vi "MonoVu.vi"() -> ()   [LabVIEW 2025]
doc: "Sequence Program with the Message Handling Queue (MHQ) for the National High Magnetic Field Laboratory in Tallahassee, Florida. \nOnce you understand how the programs works, you should be able to modify this program easily. If you have any questions, contact Minseong Lee(ml10k@my.fsu.edu), who first made this program in June, 2015."
uses:
  <vilib>/printing/OpenHTMLReport.llb/Open HTML Report in Browser (Path).vi
  <vilib>/Utility/NIReport.llb/NI_ReportGenerationCore.lvlib
panel:
  out "Row":i32=14
  in  "reset\ncursor":bool
  in  "Tab Control":T1(tab)
  in  "Sequence":i32[](listbox)=[8]
  in  "Commands":string(tree)="Remarks"
  out "Sequence Status":string="Status window"
  in  "index":i32[](listbox)=[8] caption="Sequence"
  in  "Use absolute sequence path":bool
  in  "Sequences folder path":path=path "c:/Users/user/Desktop/Sequences"
  in  "Magnet PS":u16(ring)=3 items=["Resistive Magnet", "SCM2", "SCM1", "Generic SC power supply", "PPMS"]
  in  "platform":u16(ring) items=["Mac", "PC"]
  in  "NML Data Acquisition VI":string(combo)="NML Data Acquisition-New.vi"
  in  "wait after each line executed (ms)":u32
  in  "interval in a looped execution":u32=100
  in  "PS Control VI Name":string="PS Control.vi"
  in  "override command error":bool
  in  "horizontal lines":bool
  in  "line numbers":bool
  out "most recent error":errorcluster={"status"=TRUE, "code"=1004, "source"="Open VI Reference in Get_Vi_Data.vi->WaitForAnyVI.vi->MonoVu.vi<APPEND>\nTo load a VI into memory with the Open VI Reference function, a path must be wired for the VI Path input.\n\nVI Name: <b>BLM_ManualControl.vi</b>"}
  out "execution count":i32=1
  out "macro line":i32
  out "sequence contents":string[](array[string])=["----------    AH Bridge: Set data and Time (To remove 'RTC WAS RESET' message)  ", "Write to VISA, GPIB0::27::INSTR, STORE DATE 2020,1,27", "Write to VISA, GPIB0::27::INSTR, STORE TIME 12, 45, 27", "----------    AH Bridge: Save GPIB address   ", "Write to VISA, GPIB::27::INSTR, FILE STORE GPIB USERPON", "----------    LakeShore 340 controller: change heater power (0-5, 0: off)  ", "Write to VISA, GPIB::12::INSTR, RANGE 0", "----------    Scheduled T-control for the He3 system   ", "Wait for 12 hour", "Set Temperature LS336 ( GPIB0::12::INSTR ) 45 K at 0 K/min, Output 1", "Wait for 60 s", "Wait for Temperature Less than 1.8 K Sensor C of LS336 ( GPIB0::14::INSTR ) Timeout 30 min", "Wait for 60 min", "Set Temperature LS336 ( GPIB0::12::INSTR ) 0.1 K at 0 K/min, Output 1", "----------    Motor control (use Instrumet:Set:MotorControl command structure)  ", "Set MotorControl ( BLM ) 12345 0.2", "Wait for VI value localhost, BLM_ManualControl.vi, BLM Position, Within, 12345, 10 min", "END SEQUENCE"]
  in  "error\ncheck":bool
  in  "exec window":bool caption="command window"
  in  "loop stop":bool
  in  "error \nindicator":bool
  out "Error/\nwarning?":bool
  in  "sequence utility":bool caption="seq\n utility"
  out "macro cmd no":i32=34
  in  "track \nseq.":bool
  in  "help":bool caption="Help"
  out "Buffer Edit":string[](array[string])=["----------    AH Bridge: Save GPIB address   "]
  out "Path":path=path "/Users/Shared/NML Data Acquisition/monovu/sequence templates/system typical 2.txt"
  out "Buffer History":string[](array[string])
  in  "Skip Button":bool caption="Skip"
  in  "error in (no error)":errorcluster
  in  "New Button":bool caption="New"
  in  "Program Stop":bool=TRUE caption="Program \nStop"
  in  "Save Button":bool caption="Save"
  in  "Sequence_Stop":bool caption="Stop"
  in  "Pause Button":bool caption="Pause"
  in  "Run Sequence":bool caption="Run"
  in  "Save As Button":bool caption="Save As"
  out "Cursor Position":i32=8
  out "Current Line":i32
  in  "Open Button":bool caption="Open"
  # "Timing parameters"
  # "User interface settings"
  # "Sequence Window"
  # "*"
  # "(when abs. path not used)"
  # "(bypass command syntax error)"
  # "*"
  # ": Needs to restart this VI to make the change effective"
  # "(see logbook for previous errors)"
  # "Note \n(1) For commands with timed or conditioned wait, 'go to next line' command will be executed when a certain condition is met.\n(2) For non-wait command (send command to instruments or VI without waiting response), 'go to next line' is executed automatically.\n(3) For example, 'wait for temperature command' executes repeatedly until the temperature condition is met. The visa reference will be open and closed every time it is executed.\n** Exception: 'Wait for VI value' uses a loop to use the VI reference. The loop condition has to be programmatically reset for the user intervention (skip, pause, stop) accordingly.\n\n\n\nNote for coding\n1. Each comand in the sequence line is executed repeatedly until a 'go to next line' command is executed by itself or by user interruption.\n2. 'go to next line' condition is defined in the VI of each command.\n3. Right mouse click button menu modification : Right mouse click on the sequence window -> advanced -> Run time shorcut menu -> edit"
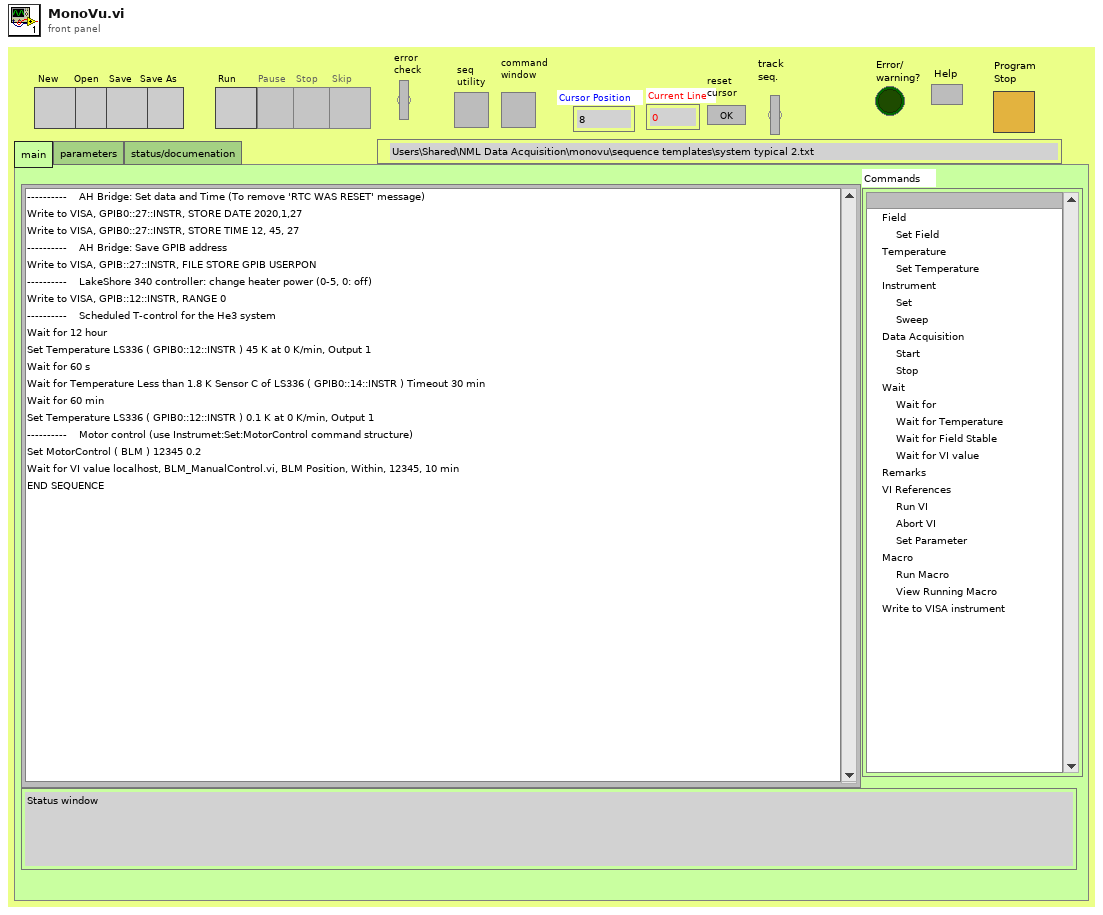
[diagram p1: front panel]
types:
  T1 = enum32{"main", "parameters", "status/documenation"}
  T2 = cluster{"Sequence_Run":refnum<vi>, "Sequence_Pause":refnum<vi>, "Sequence_Stop":refnum<vi>, "Sequence_Skip":refnum<vi>, "Program Stop":refnum<vi>, "Sequence":refnum<vi>, "NML Data Acquisition VI":refnum<vi>}
  T3 = cluster{"number of line":i32, "Signal":bool, "Command":string, "Sequence Reference":refnum<vi>, "Add or modification":bool}
  T4 = cluster{"No. of command":i32, "Parameters":string[], "Address":refnum<visa-resource-name>, "Boolean":bool, "No. of line":i32, "Initial Time":timestamp, "Current Time":timestamp, "Status":string, "Sequence Ref.":refnum<vi>, "Temp_Check":i32, "Sequence_History":string, "Subsequence":string[]}
  T5 = typedef "Command_Message.ctl" = cluster{"No. of command":i32, "Parameters":string[], "Address":refnum<visa-resource-name>, "Boolean":bool, "No. of line":i32, "Initial Time":timestamp, "Current Time":timestamp, "Status":string, "Sequence Ref.":refnum<vi>, "Temp check":i32, "Sequence_History":string, "Subsequence":string[]}
  T6 = typedef "eventsource.ctl" = u32
  T7 = typedef "Button_Reference.ctl" = cluster{"Sequence_Run":refnum<vi>, "Sequence_Pause":refnum<vi>, "Sequence_Stop":refnum<vi>, "Sequence_Skip":refnum<vi>, "Program Stop":refnum<vi>, "Sequence":refnum<vi>, "NML Data Acquisition VI":refnum<vi>}
  T8 = typedef "Command_Queue.ctl" = refnum<queue>
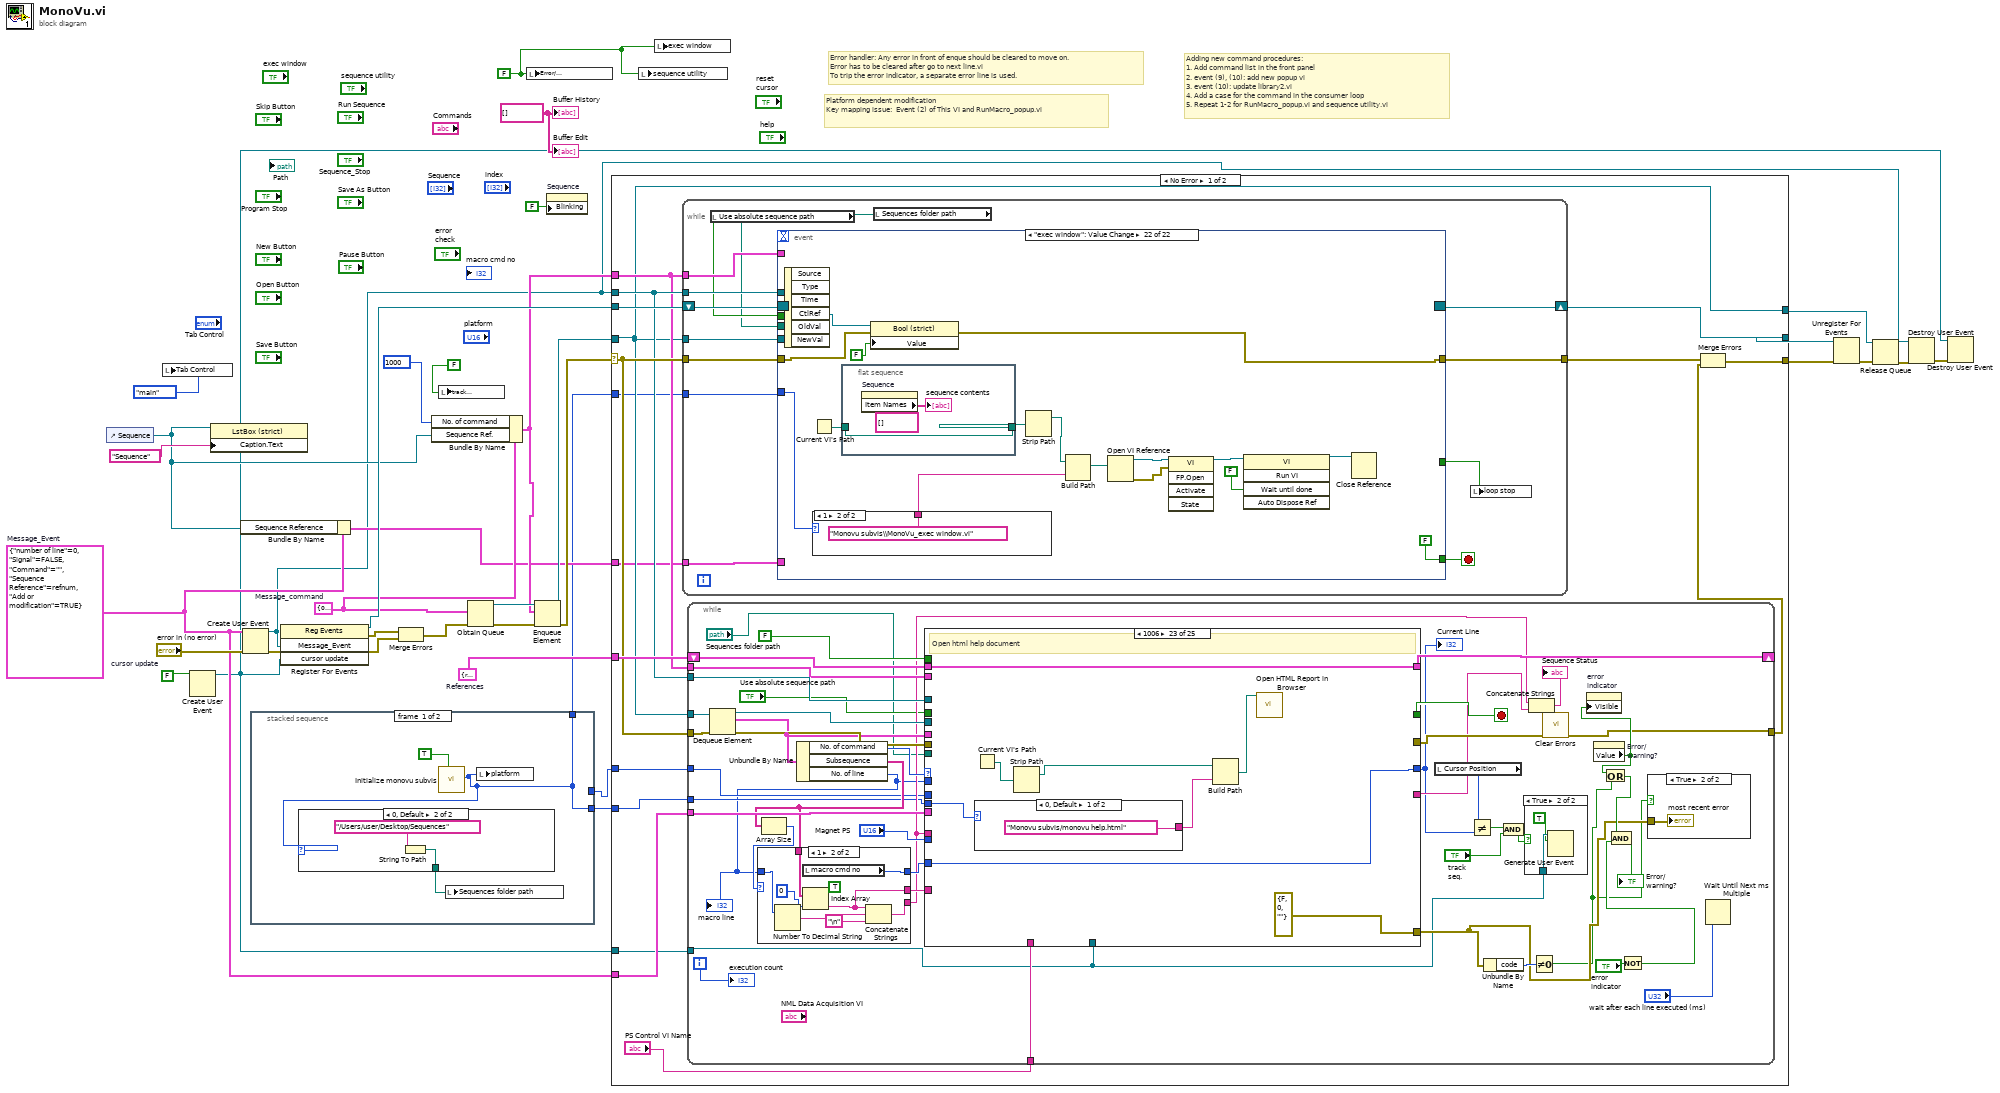
[diagram p0: block diagram]
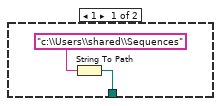
[diagram p2: hidden frame]
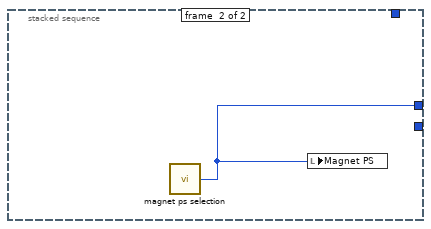
[diagram p3: hidden frame]
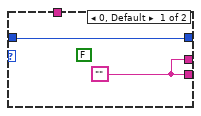
[diagram p6: hidden frame]
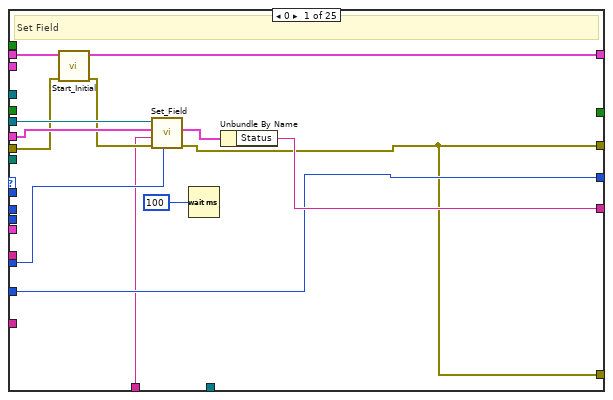
[diagram p7: hidden frame]
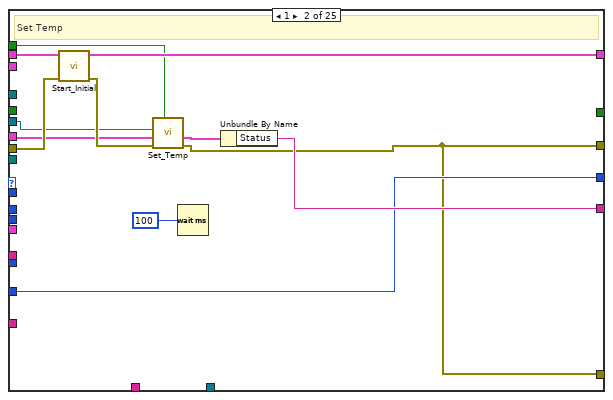
[diagram p8: hidden frame]
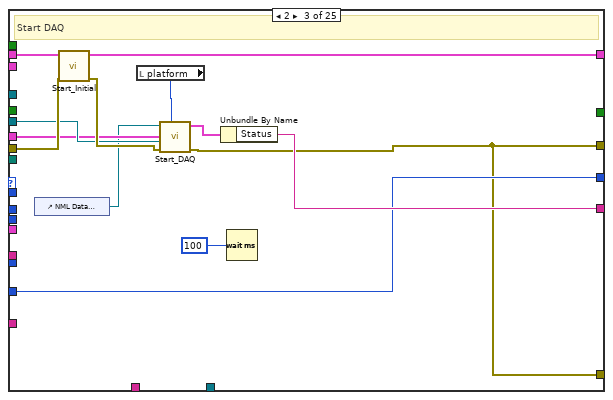
[diagram p9: hidden frame]
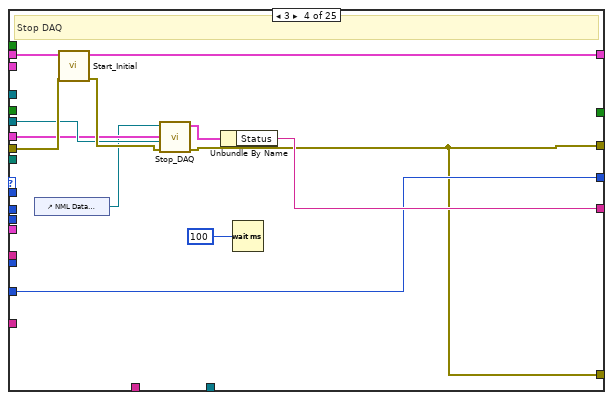
[diagram p10: hidden frame]
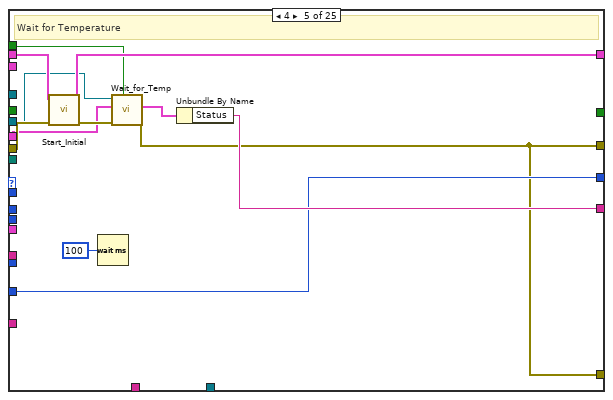
[diagram p11: hidden frame]
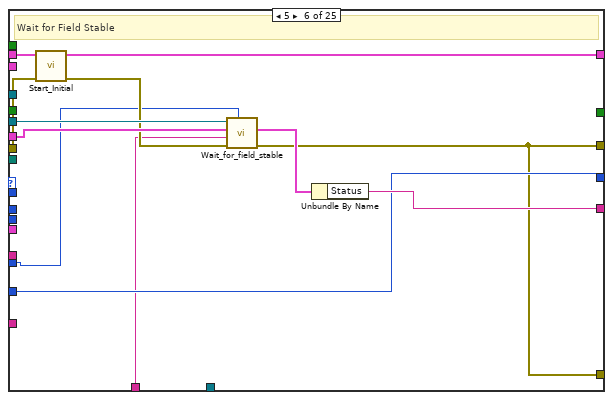
[diagram p12: hidden frame]
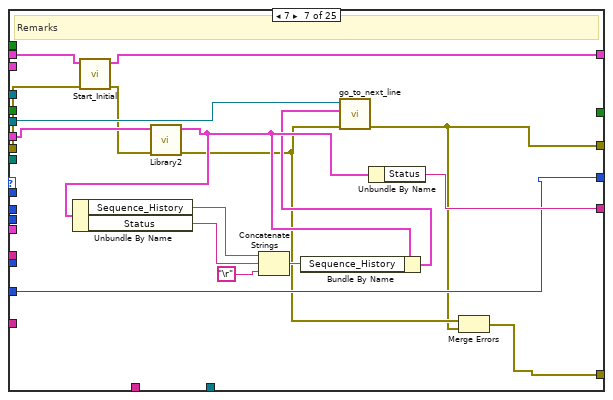
[diagram p13: hidden frame]
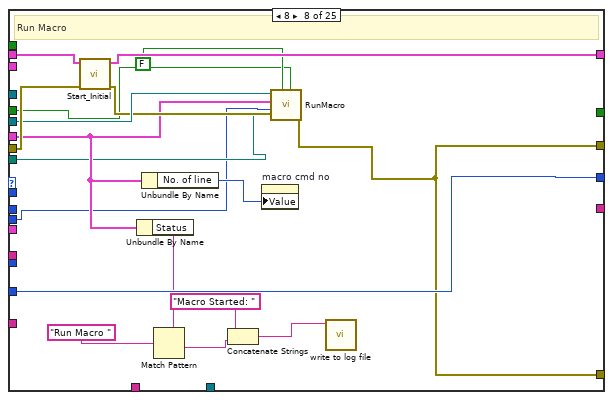
[diagram p14: hidden frame]
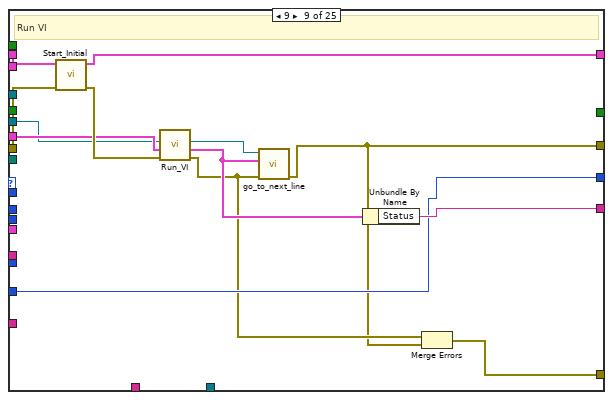
[diagram p15: hidden frame]
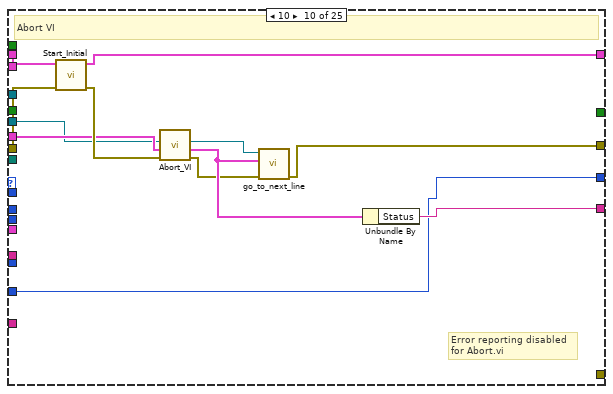
[diagram p16: hidden frame]
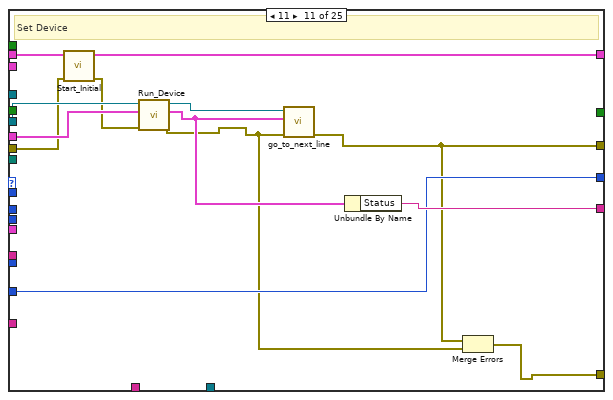
[diagram p17: hidden frame]
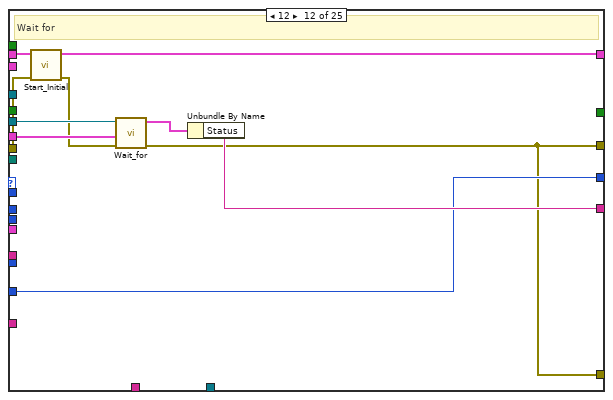
[diagram p18: hidden frame]
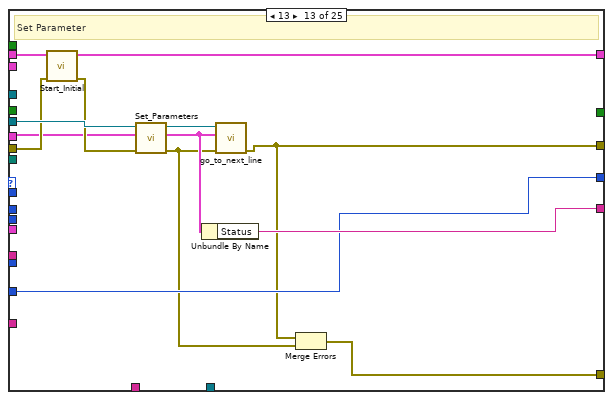
[diagram p19: hidden frame]
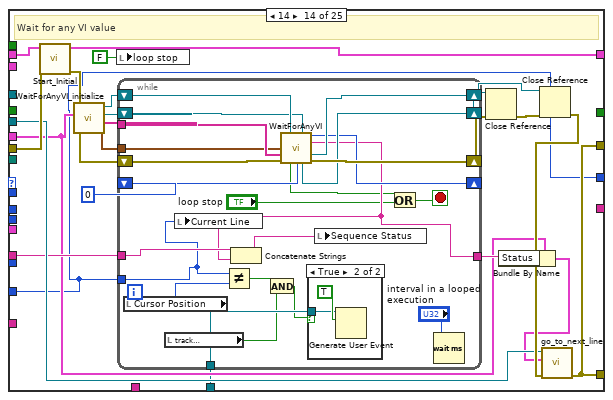
[diagram p20: hidden frame]
diagram:
  w9 = FALSE  # cursor update
  w1 = FALSE ("Error?")
  w25 = T2 {"Sequence_Run"=refnum, "Sequence_Pause"=refnum, "Sequence_Stop"=refnum, "Sequence_Skip"=refnum, "Program Stop"=refnum, "Sequence"=refnum, "NML Data Acquisition VI"=refnum}  # References
  w13 = string[] []
  w19 = T3 {"number of line"=0, "Signal"=FALSE, "Command"="", "Sequence Reference"=refnum, "Add or modification"=TRUE}  # Message_Event
  w26 = T4 {"No. of command"=0, "Parameters"=[], "Address"="", "Boolean"=TRUE, "No. of line"=0, "Initial Time"=timestamp(0 s since 1904-01-01), "Current Time"=timestamp(0 s since 1904-01-01), "Status"="", "Sequence Ref."=refnum, "Temp_Check"=0, "Sequence_History"="", "Subsequence"=[]}  # Message_command
  # "Error handler: Any error in front of enque should be cleared to move on.\nError has to be cleared after go to next line.vi\nTo trip the error indicator, a separate error line is used."
  # "Platform dependent modification\nKey mapping issue:  Event (2) of This VI and RunMacro_popup.vi"
  # "Adding new command procedures: \n1. Add command list in the front panel\n2. event (9), (10): add new popup vi\n3. event (10): update library2.vi \n4. Add a case for the command in the consumer loop\n5. Repeat 1-2 for RunMacro_popup.vi and sequence utility.vi"
  n1 = control-ref of="Sequence"() -> (w14:refnum<vi>)
  n2 = local write "Tab Control"(T1."main" ("Tab Control")) -> ()
  n3 = Create User Event(user event datatype=w9) -> (user event=w5:refnum<user-event>)  [unwired: 1 in, 1 out]
  n4 = property class="LstBox (strict)"(reference=w14, "Caption.Text"="Sequence") -> ()  [unwired: 1 in, 2 out]
  n5 = Bundle By Name(cluster=w19, "Sequence Reference"=w14) -> (w18:T3)
  n6 = Create User Event(user event datatype=w19, error in="error in (no error)") -> (user event=w6:refnum<user-event>, error out=w32:errorcluster)
  n7 = stacked-sequence {
    tunnel: [_ w42] -> w10
    tunnel: [w35 _] -> w11
    tunnel: [w35 _] -> w3
    frame #0 {
      n8 = call "Initialize monovu subvis.vi"("auto detect"=TRUE) -> ("platform used"=w35:u16)  [unwired: 8 in, 2 out]
      n9 = case shown="0, Default" w35 {
        tunnel: [w38 w41] -> w36
        frame 1 {
          n10 = String To Path(string="c:\\Users\\shared\\Sequences") -> (path=w38:path)
        }
        frame 0, Default {
          n11 = String To Path(string="/Users/user/Desktop/Sequences") -> (path=w41:path)
        }
      }
      n12 = local write "Sequences folder path"(w36) -> ()
      n13 = local write "platform"(w35) -> ()
    }
    frame #1 {
      n14 = call "magnet ps selection.vi"() -> ("Magnet PS"=w42:u16)  [unwired: 1 in]
      n15 = local write "Magnet PS"(w42) -> ()
    }
  }
  n16 = register-events(w6, w5) -> (reference out=w34:refnum<event-registration>, error out=w31:errorcluster)  [unwired: 2 in]
  n17 = Merge Errors(w31, w32) -> (w16:errorcluster)
  n18 = Bundle By Name(cluster=w26, "No. of command"=1000, "Sequence Ref."=w14) -> (w24:T4)
  n19 = local write "track \nseq."(FALSE ("track \nseq.")) -> ()
  n20 = Obtain Queue(element data type=w26, error in (no error)=w16) -> (queue out=w30:refnum<queue>, error out=w28:errorcluster)  [unwired: 3 in, 1 out]
  n21 = local write "Error/\nwarning?"(w1) -> ()
  n22 = Enqueue Element(queue=w30, element=w24, error in (no error)=w28) -> (queue out=w29:refnum<queue>, error out=w27:errorcluster)  [unwired: 1 in, 1 out]
  n23 = property on="Sequence" class="LstBox (strict)"("Blinking"=FALSE) -> ()  [unwired: 2 in, 2 out]
  n24 = case shown="No Error" w27 {
    selector: w27 -> [w56 w1456]
    tunnel: w29 -> [w52 w1454]
    tunnel: [w58 w1456] -> w21
    tunnel: w6 -> [w55 _]
    tunnel: w34 -> [w59 w1455]
    tunnel: w25 -> [w57 _]
    tunnel: w24 -> [w53 _]
    tunnel: w19 -> [w54 _]
    tunnel: [w52 w1454] -> w23
    tunnel: [w50 w1455] -> w22
    tunnel: w18 -> [w48 _]
    tunnel: w10 -> [w46 _]
    tunnel: w11 -> [w47 _]
    tunnel: w5 -> [w45 _]
    tunnel: w3 -> [w43 _]
    frame No Error {
      n25 = while {
        tunnel: w52 -> [w538]
        tunnel: w55 -> [w537]
        tunnel: w56 -> [w536]
        tunnel: [w535] -> w51
        tunnel: w53 -> [w534]
        shift-right: [w533] -> w50
        shift-left: w59 -> [w540]
        tunnel: w48 -> [w532]
        tunnel: w47 -> [w531]
        stop <- w539 stop-if-true
        # "Event_Handler"
        n26 = local read "Use absolute sequence path"() -> (w529:bool)
        n27 = local read "Sequences folder path"() -> (w528:path)
        n28 = event shown="[21] \"exec window\": Value Change" {
          selector: w540 -> [_ _ _ _ _ _ _ _ _ _ _ _ _ _ _ _ _ _ _ _ _ _]
          dyn-events: [_ _ _ _ _ _ _ _ _ _ _ _ _ _ _ _ _ _ _ _ _ _] -> w533
          timeout: _ -> [_ _ _ _ _ _ _ _ _ _ _ _ _ _ _ _ _ _ _ _ _ _]
          tunnel: [FALSE ("NewVal") FALSE ("NewVal") FALSE ("NewVal") FALSE ("NewVal") FALSE ("NewVal") FALSE ("NewVal") FALSE ("NewVal") FALSE ("NewVal") FALSE ("NewVal") FALSE ("NewVal") FALSE ("NewVal") _ FALSE ("NewVal") FALSE ("NewVal") FALSE ("NewVal") FALSE ("NewVal") FALSE ("NewVal") w1410 FALSE ("NewVal") TRUE ("NewVal") _ FALSE ("NewVal")] -> w539
          tunnel: w538 -> [w544 _ _ _ _ _ _ _ _ _ _ _ _ w1348 _ w1389 w1404 w1405 w1413 _ _ _]
          tunnel: w537 -> [w548 _ w745 w873 _ _ _ _ _ w1053 w1188 _ _ _ _ _ _ _ _ _ _ _]
          tunnel: w536 -> [w547 w573 w746 w875 w905 w943 w957 w988 w1015 w1055 w1196 _ w1339 w1347 _ w1387 w1403 w1406 w1414 w1420 w1429 w1447]
          tunnel: [w543 w561 w744 w874 w904 w941 w956 w987 w1014 w1050 w1184 _ w1339 w1343 _ w1392 w1399 w1411 w1418 w1420 w1427 w1446] -> w535
          tunnel: w534 -> [w545 w572 _ _ _ _ _ _ _ _ w1198 _ _ w1346 _ w1393 w1402 w1409 w1417 _ _ _]
          tunnel: w532 -> [_ _ w747 w872 _ _ _ _ _ w1048 w1189 _ _ _ _ _ _ _ _ _ _ _]
          tunnel: w531 -> [_ _ w741 _ _ _ _ _ _ w1039 w1172 _ _ _ _ _ _ _ _ _ w1432 w1437]
          tunnel: [_ _ _ _ _ _ _ _ _ _ _ _ _ w1341 _ TRUE ("loop stop") TRUE ("loop stop") _ _ _ _ _] -> w530
          tunnel: w529 -> [_ _ _ _ _ _ _ _ _ w1040 w1174 _ _ _ _ _ _ _ _ _ _ _]
          tunnel: w528 -> [_ _ _ _ _ _ _ _ _ w1038 w1173 _ _ _ _ _ _ _ _ _ _ _]
          event "Run Sequence": Value Change {
            n29 = event-data() -> ("NewVal"=w546:bool)  [unwired: 1 in]
            n30 = case shown="False" w546 {
              tunnel: w548 -> [_ _]
              tunnel: w547 -> [w549 w553]
              tunnel: w545 -> [_ w556]
              tunnel: w544 -> [w550 w557]
              tunnel: [w550 w552] -> _
              tunnel: [w549 w551] -> w543
              frame False {
              }
              frame True {
                n31 = Bundle By Name(cluster=w556, "No. of command"=1001) -> (w554:T4)
                n32 = Enqueue Element At Opposite End(queue=w557, element=w554, error in (no error)=w553) -> (queue out=w552:refnum<queue>, error out=w551:errorcluster)  [unwired: 1 in, 1 out]
              }
            }
            n33 = call "write to log file.vi"("input"="Run button pressed") -> ()  [unwired: 9 in, 1 out]
          }
          event User Event {
            n34 = event-data() -> ("number of line"=w571:i32, "Command"=w566:string, "Signal"=w569:bool, "Sequence Reference"=w563:refnum<vi>, "Add or modification"=w568:bool)  [unwired: 1 in]
            n35 = local read "Buffer History"() -> (w567:string[])
            n36 = local read "Buffer Edit"() -> (w565:string[])
            n37 = case shown="Default" w566 {
              selector: w566 -> [_ _ _ _ _ w697]
              tunnel: w573 -> [w580 w613 w646 w670 w694 w705]
              tunnel: [w578 w605 w637 w666 w681 w704] -> w562
              tunnel: w572 -> [_ _ _ _ _ w703]
              tunnel: w571 -> [_ _ _ _ _ w702]
              tunnel: w569 -> [_ _ _ _ _ w701]
              tunnel: w563 -> [w577 w614 w647 w671 w695 w700]
              tunnel: w568 -> [_ _ _ _ _ w699]
              tunnel: w567 -> [w579 w609 w642 _ w687 w698]
              tunnel: w565 -> [_ _ _ _ w690 _]
              tunnel: [w576 w591 w624 w654 w679 w696] -> w560
              frame "Undo" {
                # "Buffer History stores previous commands in reverse chronological order."
                n38 = Index Array(array=w579, index=0) -> (element=w587:string)
                n39 = Unflatten From String(type=w579, binary string=w587, error in (no error)=w580) -> (value=w586:string[], error out=w585:errorcluster)  [unwired: 2 in, 1 out]
                n40 = property on="Property Node" class="LstBox (strict)"(reference=w577, error in=w585, "Item Names"=w586) -> (reference out=w576:refnum<vi>, error out=w581:errorcluster)
                n41 = Delete From Array(array=w579, length=1, index=0) -> (array with subset deleted=w582:string[])  [unwired: 1 out]
                n42 = property on="Buffer History" class="Arr (strict)"(error in=w581, "Val(Sgnl)"=w582) -> (error out=w578:errorcluster)  [unwired: 1 in, 1 out]
              }
              frame "Cut" {
                n43 = property on="Property Node" class="LstBox (strict)"(reference=w614, error in=w613) -> (reference out=w611:refnum<vi>, error out=w610:errorcluster, "Item Names"=w590:string[], "Value"=w592:i32[])
                n44 = Array Size(array=w592) -> (size(s)=w603:i32)
                n45 = Index Array(array=w592, index=0) -> (element=w602:i32)
                n46 = Delete From Array(array=w590, length=w603, index=w602) -> (deleted portion=w594:string[], array with subset deleted=w596:string[])
                n47 = Array Size(array=w594) -> (size(s)=w601:i32)
                n48 = Decrement(x=w601) -> (x-1=w600:i32)
                n49 = Flatten To String(anything=w590, error in (no error)=w610) -> (data string=w607:string, error out=w606:errorcluster)  [unwired: 2 in, 1 out]
                n50 = Index Array(array=w594, index=w600) -> (element=w598:string)
                n51 = Equal?(x=w598, y="END SEQUENCE") -> (x = y?=w597:bool)
                n52 = Insert Into Array(array=w609, index=0, new element=w607) -> (w604:string[])
                n53 = case shown="True" w597 {
                  tunnel: w590 -> [_ w622]
                  tunnel: w603 -> [_ w621]
                  tunnel: w602 -> [_ w619]
                  tunnel: [w616 w618] -> w595
                  tunnel: w596 -> [w616 _]
                  tunnel: w594 -> [w615 _]
                  tunnel: [w615 w617] -> w593
                  frame False {
                  }
                  frame True {
                    n54 = Decrement(x=w621) -> (x-1=w620:i32)
                    n55 = Delete From Array(array=w622, length=w620, index=w619) -> (deleted portion=w617:string[], array with subset deleted=w618:string[])
                  }
                }
                n56 = property on="Property Node" class="LstBox (strict)"(reference=w611, error in=w606, "Item Names"=w595, "Val(Sgnl)"=w592) -> (reference out=w591:refnum<vi>, error out=w589:errorcluster)
                n57 = property on="Buffer History" class="Arr (strict)"(error in=w589, "Val(Sgnl)"=w604) -> (error out=w605:errorcluster)  [unwired: 1 in, 1 out]
                n58 = local write "Buffer Edit"(w593) -> ()
              }
              frame "Delete" {
                n59 = property on="Property Node" class="LstBox (strict)"(reference=w647, error in=w646) -> (reference out=w644:refnum<vi>, error out=w643:errorcluster, "Item Names"=w623:string[], "Value"=w625:i32[])
                n60 = Array Size(array=w625) -> (size(s)=w629:i32)
                n61 = Index Array(array=w625, index=0) -> (element=w628:i32)
                n62 = Delete From Array(array=w623, length=w629, index=w628) -> (deleted portion=w635:string[], array with subset deleted=w627:string[])
                n63 = Array Size(array=w635) -> (size(s)=w631:i32)
                n64 = Flatten To String(anything=w623, error in (no error)=w643) -> (data string=w640:string, error out=w639:errorcluster)  [unwired: 2 in, 1 out]
                n65 = Decrement(x=w631) -> (x-1=w630:i32)
                n66 = Index Array(array=w635, index=w630) -> (element=w634:string)
                n67 = Equal?(x=w634, y="END SEQUENCE") -> (x = y?=w632:bool)
                n68 = Insert Into Array(array=w642, index=0, new element=w640) -> (w636:string[])
                n69 = case shown="True" w632 {
                  tunnel: w623 -> [_ w653]
                  tunnel: w629 -> [_ w652]
                  tunnel: w628 -> [_ w650]
                  tunnel: [w648 w649] -> w626
                  tunnel: w627 -> [w648 _]
                  frame False {
                  }
                  frame True {
                    n70 = Decrement(x=w652) -> (x-1=w651:i32)
                    n71 = Delete From Array(array=w653, length=w651, index=w650) -> (array with subset deleted=w649:string[])  [unwired: 1 out]
                  }
                }
                n72 = property on="Property Node" class="LstBox (strict)"(reference=w644, error in=w639, "Item Names"=w626, "Val(Sgnl)"=w625) -> (reference out=w624:refnum<vi>, error out=w638:errorcluster)
                n73 = property on="Buffer History" class="Arr (strict)"(error in=w638, "Val(Sgnl)"=w636) -> (error out=w637:errorcluster)  [unwired: 1 in, 1 out]
              }
              frame "Copy" {
                n74 = property on="Property Node" class="LstBox (strict)"(reference=w671, error in=w670) -> (reference out=w668:refnum<vi>, error out=w667:errorcluster, "Item Names"=w656:string[], "Value"=w655:i32[])
                n75 = Array Size(array=w655) -> (size(s)=w660:i32)
                n76 = Index Array(array=w655, index=0) -> (element=w659:i32)
                n77 = Array Subset(array=w656, index=w659, length=w660) -> (w658:string[])
                n78 = Array Size(array=w658) -> (size(s)=w665:i32)
                n79 = Decrement(x=w665) -> (x-1=w664:i32)
                n80 = property on="Property Node" class="LstBox (strict)"(reference=w668, error in=w667, "Item Names"=w656, "Val(Sgnl)"=w655) -> (reference out=w654:refnum<vi>, error out=w666:errorcluster)
                n81 = Index Array(array=w658, index=w664) -> (element=w663:string)
                n82 = Equal?(x=w663, y="END SEQUENCE") -> (x = y?=w661:bool)
                n83 = case shown="True" w661 {
                  tunnel: w660 -> [_ w677]
                  tunnel: w659 -> [_ w675]
                  tunnel: [w672 w673] -> w657
                  tunnel: w658 -> [w672 _]
                  tunnel: w656 -> [_ w674]
                  frame False {
                  }
                  frame True {
                    n84 = Decrement(x=w677) -> (x-1=w676:i32)
                    n85 = Delete From Array(array=w674, length=w676, index=w675) -> (deleted portion=w673:string[])  [unwired: 1 out]
                  }
                }
                n86 = local write "Buffer Edit"(w657) -> ()
              }
              frame "Paste" {
                n87 = property on="Property Node" class="LstBox (strict)"(reference=w695, error in=w694) -> (reference out=w692:refnum<vi>, error out=w684:errorcluster, "Item Names"=w678:string[], "Value"=w680:i32[])
                n88 = Index Array(array=w680, index=0) -> (element=w691:i32)
                n89 = Insert Into Array(array=w678, index=w691, new element=w690) -> (w688:string[])
                n90 = Flatten To String(anything=w678, error in (no error)=w684) -> (data string=w689:string, error out=w683:errorcluster)  [unwired: 2 in, 1 out]
                n91 = property on="Property Node" class="LstBox (strict)"(reference=w692, error in=w683, "Item Names"=w688, "Val(Sgnl)"=w680) -> (reference out=w679:refnum<vi>, error out=w682:errorcluster)
                n92 = Insert Into Array(array=w687, index=0, new element=w689) -> (w685:string[])
                n93 = property on="Buffer History" class="Arr (strict)"(error in=w682, "Val(Sgnl)"=w685) -> (error out=w681:errorcluster)  [unwired: 1 in, 1 out]
              }
              frame Default {
                n94 = case shown="False" w699 {
                  tunnel: w705 -> [w723 w739]
                  tunnel: [w708 w726] -> w704
                  tunnel: w703 -> [_ _]
                  tunnel: w702 -> [_ _]
                  tunnel: w701 -> [_ _]
                  tunnel: w700 -> [w722 w738]
                  tunnel: w697 -> [w721 w737]
                  tunnel: w698 -> [w720 w736]
                  tunnel: [w710 w728] -> w696
                  frame True {
                    n95 = property class="LstBox (strict)"(reference=w722, error in=w723) -> (reference out=w718:refnum<vi>, error out=w714:errorcluster, "Item Names"=w715:string[], "Value"=w711:i32[])
                    n96 = Index Array(array=w711, index=0) -> (element=w709:i32)
                    n97 = Flatten To String(anything=w715, error in (no error)=w714) -> (data string=w716:string, error out=w707:errorcluster)  [unwired: 2 in, 1 out]
                    n98 = Insert Into Array(array=w715, index=w709, new element=w721) -> (w717:string[])
                    n99 = Insert Into Array(array=w720, index=0, new element=w716) -> (w712:string[])
                    n100 = property on="Buffer History" class="Arr (strict)"(error in=w707, "Val(Sgnl)"=w712) -> (error out=w706:errorcluster)  [unwired: 1 in, 1 out]
                    n101 = property class="LstBox (strict)"(reference=w718, error in=w706, "Item Names"=w717, "Value"=w711) -> (reference out=w710:refnum<vi>, error out=w708:errorcluster)
                  }
                  frame False {
                    n102 = property class="LstBox (strict)"(reference=w738, error in=w739) -> (reference out=w735:refnum<vi>, error out=w731:errorcluster, "Item Names"=w732:string[])
                    n103 = local read "Row"() -> (w727:i32)
                    n104 = Flatten To String(anything=w732, error in (no error)=w731) -> (data string=w734:string, error out=w725:errorcluster)  [unwired: 2 in, 1 out]
                    n105 = Replace Array Subset(array=w732, new element=w737, index=w727) -> (w733:string[])
                    n106 = Insert Into Array(array=w736, index=0, new element=w734) -> (w729:string[])
                    n107 = property on="Buffer History" class="Arr (strict)"(error in=w725, "Val(Sgnl)"=w729) -> (error out=w724:errorcluster)  [unwired: 1 in, 1 out]
                    n108 = property class="LstBox (strict)"(reference=w735, error in=w724, "Item Names"=w733) -> (reference out=w728:refnum<vi>, error out=w726:errorcluster)
                  }
                }
              }
            }
            n109 = property class="LstBox (strict)"(reference=w560, error in=w562) -> (error out=w561:errorcluster, "Item Names"=w559:string[])  [unwired: 1 out]
            n110 = Array Size(array=w559) -> (size(s)=w558:i32)
            n111 = for {
              N: w558 -> [_]
              tunnel: [w574] -> w564 mode=indexing
              i -> [w575]
              n112 = Number To Decimal String(number=w575) -> (decimal integer string=w574:string)  [unwired: 1 in]
            }
            n113 = property on="index" class="LstBox (strict)"("Item Names"=w564) -> ()  [unwired: 2 in, 2 out]
          }
          event "Sequence": Key Down {
            # "PC (1):\nDelete:  83\nundo: 44\ncut: 45\ncopy: 46\npaste: 47"
            # "Mac (0)\nDelete:  117\nundo: 6\ncut: 7\ncopy: 8\npaste: 9"
            n114 = event-data() -> ("ScanCode"=w748:i16, "PlatMods.Ctrl"=w742:bool, "PlatMods.Shift"=w740:bool)  [unwired: 1 in]
            n115 = case shown="1" w741 {
              tunnel: w748 -> [w754 w815]
              tunnel: w747 -> [w753 w814]
              tunnel: w746 -> [w752 w813]
              tunnel: w745 -> [w751 w812]
              tunnel: [w750 w811] -> w744
              tunnel: w742 -> [_ w810]
              tunnel: w740 -> [w749 _]
              frame 1 {
                n116 = case shown="44" w754 {
                  tunnel: w753 -> [_ w760 w763 w775 w787 w799]
                  tunnel: w752 -> [w755 w758 w765 w777 w789 w801]
                  tunnel: w751 -> [_ w757 w762 w774 w786 w798]
                  tunnel: [w755 w756 w764 w776 w788 w800] -> w750
                  tunnel: w749 -> [_ _ w766 w778 w790 w802]
                  frame 0, Default {
                  }
                  frame 83 {
                    n117 = Bundle By Name(cluster=w760, "Command"="Delete") -> (w759:T3)
                    n118 = Generate User Event(user event=w757, event data cluster=w759, error in=w758) -> (error out=w756:errorcluster)  [unwired: 1 in, 1 out]
                  }
                  frame 44 {
                    n119 = case shown="True" w766 {
                      tunnel: w765 -> [w767 w769]
                      tunnel: [w767 w771] -> w764
                      tunnel: w763 -> [_ w770]
                      tunnel: w762 -> [_ w768]
                      frame False {
                      }
                      frame True {
                        n120 = Bundle By Name(cluster=w770, "Command"="Undo") -> (w772:T3)
                        n121 = Generate User Event(user event=w768, event data cluster=w772, error in=w769) -> (error out=w771:errorcluster)  [unwired: 1 in, 1 out]
                      }
                    }
                  }
                  frame 45 {
                    n122 = case shown="True" w778 {
                      tunnel: w777 -> [w779 w781]
                      tunnel: [w779 w783] -> w776
                      tunnel: w775 -> [_ w782]
                      tunnel: w774 -> [_ w780]
                      frame False {
                      }
                      frame True {
                        n123 = Bundle By Name(cluster=w782, "Command"="Cut") -> (w784:T3)
                        n124 = Generate User Event(user event=w780, event data cluster=w784, error in=w781) -> (error out=w783:errorcluster)  [unwired: 1 in, 1 out]
                      }
                    }
                  }
                  frame 46 {
                    n125 = case shown="True" w790 {
                      tunnel: w789 -> [w791 w793]
                      tunnel: [w791 w795] -> w788
                      tunnel: w787 -> [_ w794]
                      tunnel: w786 -> [_ w792]
                      frame False {
                      }
                      frame True {
                        n126 = Bundle By Name(cluster=w794, "Command"="Copy") -> (w796:T3)
                        n127 = Generate User Event(user event=w792, event data cluster=w796, error in=w793) -> (error out=w795:errorcluster)  [unwired: 1 in, 1 out]
                      }
                    }
                  }
                  frame 47 {
                    n128 = case shown="True" w802 {
                      tunnel: w801 -> [w803 w805]
                      tunnel: [w803 w807] -> w800
                      tunnel: w799 -> [_ w806]
                      tunnel: w798 -> [_ w804]
                      frame False {
                      }
                      frame True {
                        n129 = Bundle By Name(cluster=w806, "Command"="Paste") -> (w808:T3)
                        n130 = Generate User Event(user event=w804, event data cluster=w808, error in=w805) -> (error out=w807:errorcluster)  [unwired: 1 in, 1 out]
                      }
                    }
                  }
                }
              }
              frame 0, Default {
                n131 = case shown="6" w815 {
                  tunnel: w814 -> [_ w821 w824 w836 w848 w860]
                  tunnel: w813 -> [w816 w819 w826 w838 w850 w862]
                  tunnel: w812 -> [_ w818 w823 w835 w847 w859]
                  tunnel: [w816 w817 w825 w837 w849 w861] -> w811
                  tunnel: w810 -> [_ _ w827 w839 w851 w863]
                  frame 0, Default {
                  }
                  frame 117 {
                    n132 = Bundle By Name(cluster=w821, "Command"="Delete") -> (w820:T3)
                    n133 = Generate User Event(user event=w818, event data cluster=w820, error in=w819) -> (error out=w817:errorcluster)  [unwired: 1 in, 1 out]
                  }
                  frame 6 {
                    n134 = case shown="True" w827 {
                      tunnel: w826 -> [w828 w830]
                      tunnel: [w828 w832] -> w825
                      tunnel: w824 -> [_ w831]
                      tunnel: w823 -> [_ w829]
                      frame False {
                      }
                      frame True {
                        n135 = Bundle By Name(cluster=w831, "Command"="Undo") -> (w833:T3)
                        n136 = Generate User Event(user event=w829, event data cluster=w833, error in=w830) -> (error out=w832:errorcluster)  [unwired: 1 in, 1 out]
                      }
                    }
                  }
                  frame 7 {
                    n137 = case shown="True" w839 {
                      tunnel: w838 -> [w840 w842]
                      tunnel: [w840 w844] -> w837
                      tunnel: w836 -> [_ w843]
                      tunnel: w835 -> [_ w841]
                      frame False {
                      }
                      frame True {
                        n138 = Bundle By Name(cluster=w843, "Command"="Cut") -> (w845:T3)
                        n139 = Generate User Event(user event=w841, event data cluster=w845, error in=w842) -> (error out=w844:errorcluster)  [unwired: 1 in, 1 out]
                      }
                    }
                  }
                  frame 8 {
                    n140 = case shown="True" w851 {
                      tunnel: w850 -> [w852 w854]
                      tunnel: [w852 w856] -> w849
                      tunnel: w848 -> [_ w855]
                      tunnel: w847 -> [_ w853]
                      frame False {
                      }
                      frame True {
                        n141 = Bundle By Name(cluster=w855, "Command"="Copy") -> (w857:T3)
                        n142 = Generate User Event(user event=w853, event data cluster=w857, error in=w854) -> (error out=w856:errorcluster)  [unwired: 1 in, 1 out]
                      }
                    }
                  }
                  frame 9 {
                    n143 = case shown="True" w863 {
                      tunnel: w862 -> [w864 w866]
                      tunnel: [w864 w868] -> w861
                      tunnel: w860 -> [_ w867]
                      tunnel: w859 -> [_ w865]
                      frame False {
                      }
                      frame True {
                        n144 = Bundle By Name(cluster=w867, "Command"="Paste") -> (w869:T3)
                        n145 = Generate User Event(user event=w865, event data cluster=w869, error in=w866) -> (error out=w868:errorcluster)  [unwired: 1 in, 1 out]
                      }
                    }
                  }
                }
              }
            }
          }
          event "Sequence": Shortcut Menu Selection (User) {
            n146 = event-data() -> ("ItemTag"=w876:string)  [unwired: 1 in]
            n147 = case shown="\"Undo\"" w876 {
              selector: w876 -> [_ w881 w887 w893 w899]
              tunnel: w875 -> [w877 w879 w885 w891 w897]
              tunnel: [w877 w878 w884 w890 w896] -> w874
              tunnel: w873 -> [_ w883 w889 w895 w901]
              tunnel: w872 -> [_ w882 w888 w894 w900]
              frame Default {
              }
              frame "Undo" {
                n148 = Bundle By Name(cluster=w882, "Command"=w881) -> (w880:T3)
                n149 = Generate User Event(user event=w883, event data cluster=w880, error in=w879) -> (error out=w878:errorcluster)  [unwired: 1 in, 1 out]
              }
              frame "Cut" {
                n150 = Bundle By Name(cluster=w888, "Command"=w887) -> (w886:T3)
                n151 = Generate User Event(user event=w889, event data cluster=w886, error in=w885) -> (error out=w884:errorcluster)  [unwired: 1 in, 1 out]
              }
              frame "Copy" {
                n152 = Bundle By Name(cluster=w894, "Command"=w893) -> (w892:T3)
                n153 = Generate User Event(user event=w895, event data cluster=w892, error in=w891) -> (error out=w890:errorcluster)  [unwired: 1 in, 1 out]
              }
              frame "Paste" {
                n154 = Bundle By Name(cluster=w900, "Command"=w899) -> (w898:T3)
                n155 = Generate User Event(user event=w901, event data cluster=w898, error in=w897) -> (error out=w896:errorcluster)  [unwired: 1 in, 1 out]
              }
            }
          }
          event "New Button": Value Change {
            n156 = event-data() -> ("NewVal"=w906:bool, "CtlRef"=w903:refnum<vi>)  [unwired: 1 in]
            n157 = case shown="True" w906 {
              tunnel: w905 -> [w907 w923]
              tunnel: [w907 w915] -> w904
              tunnel: w903 -> [_ w918]
              frame False {
              }
              frame True {
                n158 = property on="Sequence" class="LstBox (strict)"(error in=w923) -> (error out=w914:errorcluster, "Caption.Text"=w922:string, "Item Names"=w919:string[])  [unwired: 1 in, 1 out]
                n159 = property on="Buffer History" class="Arr (strict)"(error in=w914) -> (error out=w913:errorcluster, "Value"=w912:string[])  [unwired: 1 in, 1 out]
                n160 = Equal?(x=w922, y="Sequence*") -> (x = y?=w920:bool)
                n161 = case shown="False" w920 {
                  tunnel: w913 -> [w928 w939]
                  tunnel: w919 -> [_ w940]
                  tunnel: [w929 w934] -> w911
                  tunnel: w918 -> [w927 w933]
                  tunnel: [w927 w933] -> w917
                  tunnel: w912 -> [_ w931]
                  tunnel: [string[] [] ("Buffer out") w930] -> w909
                  frame False {
                    n162 = property on="Sequence" class="LstBox (strict)"(error in=w928, "Item Names"=string[] ["END SEQUENCE"], "Caption.Text"="Sequence") -> (error out=w929:errorcluster)  [unwired: 1 in, 1 out]
                  }
                  frame True {
                    n163 = property on="Path" class="Path"(error in=w939) -> (error out=w938:errorcluster, "Value"=w937:path)  [unwired: 1 in, 1 out]
                    n164 = call "New_File.vi"("error in (no error)"=w938, "Path"=w937, "Buffer in"=w931, "Sequence in"=w940) -> ("error out"=w936:errorcluster, "Sequence Caption"=w932:string, "Buffer out"=w930:string[], "Sequence_out"=w935:string[])  [unwired: 4 in]
                    n165 = property on="Sequence" class="LstBox (strict)"(error in=w936, "Item Names"=w935, "Caption.Text"=w932) -> (error out=w934:errorcluster)  [unwired: 1 in, 1 out]
                  }
                }
                n166 = property on="Buffer History" class="Arr (strict)"(error in=w911, "Value"=w909) -> (error out=w910:errorcluster)  [unwired: 1 in, 1 out]
                n167 = property class="Bool (strict)"(reference=w917, error in=w910, "Value"=FALSE) -> (error out=w915:errorcluster)  [unwired: 1 out]
                n168 = property on="Sequence" class="LstBox (strict)"("Top Row"=0) -> ()  [unwired: 2 in, 2 out]
              }
            }
          }
          event "Buffer History": Value Change {
            n169 = event-data() -> ("NewVal"=w947:string[])  [unwired: 1 in]
            n170 = Array Size(array=w947) -> (size(s)=w946:i32)
            n171 = Equal?(x=w946, y=0) -> (x = y?=w944:bool)
            n172 = case shown="False" w944 {
              tunnel: w943 -> [w949 w952]
              tunnel: [w948 w951] -> w941
              frame True {
                n173 = property on="Sequence" class="LstBox (strict)"(error in=w949, "Caption.Text"="Sequence") -> (error out=w948:errorcluster)  [unwired: 1 in, 1 out]
              }
              frame False {
                n174 = property on="Sequence" class="LstBox (strict)"(error in=w952, "Caption.Text"="Sequence*") -> (error out=w951:errorcluster)  [unwired: 1 in, 1 out]
              }
            }
          }
          event "Open Button": Value Change {
            n175 = event-data() -> ("NewVal"=w958:bool, "CtlRef"=w955:refnum<vi>)  [unwired: 1 in]
            n176 = case shown="True" w958 {
              tunnel: w957 -> [w959 w982]
              tunnel: [w959 w964] -> w956
              tunnel: w955 -> [_ w967]
              frame False {
              }
              frame True {
                n177 = property on="Sequence" class="LstBox (strict)"(error in=w982) -> (error out=w978:errorcluster, "Caption.Text"=w980:string, "Item Names"=w979:string[])  [unwired: 1 in, 1 out]
                n178 = Equal?(x=w980, y="Sequence*") -> (x = y?=w968:bool)
                n179 = property on="Buffer History" class="Arr (strict)"(error in=w978) -> (error out=w976:errorcluster, "Value"=w977:string[])  [unwired: 1 in, 1 out]
                n180 = property on="Path" class="Path"(error in=w976) -> (error out=w974:errorcluster, "Value"=w975:path)  [unwired: 1 in, 1 out]
                n181 = call "Open_File.vi"("Message?"=w968, "Path in"=w975, "error in (no error)"=w974, "Sequence in"=w979, "Buffer in"=w977, "Sequence Caption in"=w980) -> ("error out"=w963:errorcluster, "Sequence out"=w961:string[], "Buffer out"=w971:string[], "Sequence Caption out"=w973:string, "Path out"=w969:path, "top row"=w962:i32)
                n182 = property on="Sequence" class="LstBox (strict)"("Top Row"=w962) -> ()  [unwired: 2 in, 2 out]
                n183 = for {
                  tunnel: w961 -> [_] mode=indexing
                  tunnel: [w983] -> w960 mode=indexing
                  i -> [w984]
                  n184 = Number To Decimal String(number=w984) -> (decimal integer string=w983:string)  [unwired: 1 in]
                }
                n185 = property on="Sequence" class="LstBox (strict)"(error in=w963, "Item Names"=w961, "Caption.Text"=w973) -> (error out=w972:errorcluster)  [unwired: 1 in, 1 out]
                n186 = property on="index" class="LstBox (strict)"("Item Names"=w960) -> ()  [unwired: 2 in, 2 out]
                n187 = property on="Buffer History" class="Arr (strict)"(error in=w972, "Value"=w971) -> (error out=w970:errorcluster)  [unwired: 1 in, 1 out]
                n188 = property on="Path" class="Path"(error in=w970, "Value"=w969) -> (error out=w966:errorcluster)  [unwired: 1 in, 1 out]
                n189 = property class="Bool (strict)"(reference=w967, error in=w966, "Value"=FALSE) -> (error out=w964:errorcluster)  [unwired: 1 out]
              }
            }
          }
          event "Save Button": Value Change {
            n190 = event-data() -> ("NewVal"=w989:bool, "CtlRef"=w986:refnum<vi>)  [unwired: 1 in]
            n191 = case shown="True" w989 {
              tunnel: w988 -> [w990 w1007]
              tunnel: [w990 w991] -> w987
              tunnel: w986 -> [_ w994]
              frame False {
              }
              frame True {
                n192 = property on="Path" class="Path"(error in=w1007) -> (error out=w1006:errorcluster, "Value"=w1009:path)  [unwired: 1 in, 1 out]
                n193 = Not Equal?(x=path "", y=w1009) -> (x != y?=w1010:bool)
                n194 = property on="Buffer History" class="Arr (strict)"(error in=w1006) -> (error out=w1005:errorcluster, "Value"=w1008:string[])  [unwired: 1 in, 1 out]
                n195 = property on="Sequence" class="LstBox (strict)"(error in=w1005) -> (error out=w1004:errorcluster, "Item Names"=w1003:string[], "Caption.Text"=w1002:string)  [unwired: 1 in, 1 out]
                n196 = call "Save_File.vi"("Sequence caption in"=w1002, "Path?"=w1010, "error in (no error)"=w1004, "Sequence in"=w1003, "Buffer in"=w1008, "Path in"=w1009) -> ("error out"=w1001:errorcluster, "Sequence out"=w997:string[], "Buffer out"=w999:string[], "Path out"=w995:path, "Sequence caption out"=w998:string)  [unwired: 1 in]
                n197 = property on="Buffer History" class="Arr (strict)"(error in=w1001, "Value"=w999) -> (error out=w1000:errorcluster)  [unwired: 1 in, 1 out]
                n198 = property on="Sequence" class="LstBox (strict)"(error in=w1000, "Item Names"=w997, "Caption.Text"=w998) -> (error out=w996:errorcluster)  [unwired: 1 in, 1 out]
                n199 = property on="Path" class="Path"(error in=w996, "Value"=w995) -> (error out=w993:errorcluster)  [unwired: 1 in, 1 out]
                n200 = property class="Bool (strict)"(reference=w994, error in=w993, "Value"=FALSE) -> (error out=w991:errorcluster)  [unwired: 1 out]
              }
            }
          }
          event "Save As Button": Value Change {
            n201 = event-data() -> ("NewVal"=w1016:bool, "CtlRef"=w1013:refnum<vi>)  [unwired: 1 in]
            n202 = case shown="True" w1016 {
              tunnel: w1015 -> [w1017 w1035]
              tunnel: [w1017 w1019] -> w1014
              tunnel: w1013 -> [_ w1022]
              frame False {
              }
              frame True {
                n203 = property on="Path" class="Path"(error in=w1035) -> (error out=w1034:errorcluster, "Value"=w1037:path)  [unwired: 1 in, 1 out]
                n204 = property on="Buffer History" class="Arr (strict)"(error in=w1034) -> (error out=w1033:errorcluster, "Value"=w1036:string[])  [unwired: 1 in, 1 out]
                n205 = property on="Sequence" class="LstBox (strict)"(error in=w1033) -> (error out=w1032:errorcluster, "Item Names"=w1031:string[], "Caption.Text"=w1030:string)  [unwired: 1 in, 1 out]
                n206 = call "Save_File.vi"("Sequence caption in"=w1030, "Path?"=FALSE, "error in (no error)"=w1032, "Sequence in"=w1031, "Buffer in"=w1036, "Path in"=w1037) -> ("error out"=w1029:errorcluster, "Sequence out"=w1025:string[], "Buffer out"=w1027:string[], "Path out"=w1023:path, "Sequence caption out"=w1026:string)  [unwired: 1 in]
                n207 = property on="Buffer History" class="Arr (strict)"(error in=w1029, "Value"=w1027) -> (error out=w1028:errorcluster)  [unwired: 1 in, 1 out]
                n208 = property on="Sequence" class="LstBox (strict)"(error in=w1028, "Item Names"=w1025, "Caption.Text"=w1026) -> (error out=w1024:errorcluster)  [unwired: 1 in, 1 out]
                n209 = property on="Path" class="Path"(error in=w1024, "Value"=w1023) -> (error out=w1021:errorcluster)  [unwired: 1 in, 1 out]
                n210 = property class="Bool (strict)"(reference=w1022, error in=w1021, "Value"=FALSE) -> (error out=w1019:errorcluster)  [unwired: 1 out]
              }
            }
          }
          event "Commands": Double Click {
            n211 = event-data() -> ("Tag"=w1054:string)  [unwired: 1 in]
            n212 = case shown="\"Write to VISA instrument\"" w1054 {
              tunnel: w1055 -> [w1069 w1075 w1081 w1087 w1093 w1099 w1105 w1111 w1117 w1123 w1129 w1135 w1138 w1143 w1151 w1159 w1160 w1165]
              tunnel: [w1069 w1073 w1078 w1085 w1090 w1096 w1102 w1108 w1114 w1120 w1126 w1132 w1138 w1143 w1148 w1154 w1162 w1168] -> w1051
              tunnel: w1053 -> [w1068 w1072 w1079 w1086 w1092 w1098 w1104 w1110 w1116 w1122 w1128 w1134 w1140 w1145 w1150 w1156 _ w1170]
              tunnel: w1039 -> [_ _ _ _ _ _ _ _ _ _ _ _ _ _ _ w1157 _ _]
              tunnel: [TRUE ("Cancel") w1074 w1080 w1084 w1091 w1097 w1103 w1109 w1115 w1121 w1127 w1133 FALSE ("Signal") FALSE ("Signal") w1149 w1155 _ w1169] -> w1043
              tunnel: [w1068 w1072 w1079 w1086 w1092 w1098 w1104 w1110 w1116 w1122 w1128 w1134 w1140 w1145 w1150 w1156 _ w1170] -> w1049
              tunnel: [_ TRUE ("Add or modification") TRUE ("Add or modification") TRUE ("Add or modification") TRUE ("Add or modification") TRUE ("Add or modification") TRUE ("Add or modification") TRUE ("Add or modification") TRUE ("Add or modification") TRUE ("Add or modification") TRUE ("Add or modification") TRUE ("Add or modification") TRUE ("Add or modification") TRUE ("Add or modification") TRUE ("Signal") TRUE ("Signal") _ TRUE ("Add or modification")] -> w1047
              tunnel: [_ w1071 w1076 w1082 w1088 w1094 w1100 w1106 w1112 w1119 w1124 w1130 "Stop" ("Command") "Wait for Field Stable" ("Command") w1146 w1152 _ w1166] -> w1045
              frame Default {
              }
              frame "Set Field" {
                n213 = call "SetField_popup.vi"("error in (no error)"=w1075) -> ("Output Line command"=w1071:string, "Cancel"=w1074:bool, "error out"=w1073:errorcluster)  [unwired: 5 in]
              }
              frame "Set Temperature" {
                n214 = call "SetTemp_popup.vi"("error in (no error)"=w1081) -> ("error out"=w1078:errorcluster, "Cancel"=w1080:bool, "Output Line Command"=w1076:string)  [unwired: 7 in]
              }
              frame "Wait for Temperature" {
                n215 = call "SetWaitForTemp_popup.vi"("error in (no error)"=w1087) -> ("Output Line Command"=w1082:string, "Cancel"=w1084:bool, "error out"=w1085:errorcluster)  [unwired: 7 in]
              }
              frame "Wait for" {
                n216 = call "SetWaitFor_popup.vi"("error in (no error)"=w1093) -> ("error out"=w1090:errorcluster, "Cancel"=w1091:bool, "Output Line Command"=w1088:string)  [unwired: 7 in]
              }
              frame "Start" {
                n217 = call "SetStart_popup.vi"("error in (no error)"=w1099) -> ("Output Line Command"=w1094:string, "Cancel"=w1097:bool, "error out"=w1096:errorcluster)  [unwired: 7 in]
              }
              frame "Remarks" {
                n218 = call "SetRemarks_popup.vi"("error in (no error)"=w1105) -> ("Cancel"=w1103:bool, "Output Line Command"=w1100:string, "error out"=w1102:errorcluster)  [unwired: 7 in]
              }
              frame "Run VI" {
                n219 = call "SetRunVI_popup.vi"("error in (no error)"=w1111) -> ("Cancel"=w1109:bool, "Output Line Command"=w1106:string, "error out"=w1108:errorcluster)  [unwired: 7 in]
              }
              frame "Abort VI" {
                n220 = call "SetAbortVI_popup.vi"("error in (no error)"=w1117) -> ("Cancel"=w1115:bool, "Output Line Command"=w1112:string, "error out"=w1114:errorcluster)  [unwired: 7 in]
              }
              frame "Set Parameter" {
                n221 = call "SetParameter_popup.vi"("error in (no error)"=w1123) -> ("error out"=w1120:errorcluster, "Cancel"=w1121:bool, "Output Line Command"=w1119:string)  [unwired: 7 in]
              }
              frame "Set" {
                n222 = call "SetDevice_popup.vi"("error in (no error)"=w1129) -> ("Cancel"=w1127:bool, "Output Line Command"=w1124:string, "error out"=w1126:errorcluster)  [unwired: 7 in]
              }
              frame "Sweep" {
                n223 = call "SetSweep_popup.vi"("error in (no error)"=w1135) -> ("Cancel"=w1133:bool, "Output Line Command"=w1130:string, "error out"=w1132:errorcluster)  [unwired: 7 in]
              }
              frame "Stop" {
              }
              frame "Wait for Field Stable" {
              }
              frame "Wait for VI value" {
                n224 = call "SetWaitForAnyVI_popup.vi"("error in (no error)"=w1151) -> ("error out"=w1148:errorcluster, "Cancel"=w1149:bool, "Output Line Command"=w1146:string)  [unwired: 7 in]
              }
              frame "Run Macro" {
                n225 = call "RunMacro_popup.vi"("load?"=FALSE, "platform"=w1157, "error in (no error)"=w1159) -> ("Cancel"=w1155:bool, "command out"=w1152:string, "error out"=w1154:errorcluster)  [unwired: 5 in]
              }
              frame "View Running Macro" {
                n226 = vi-ref "RunMacro.vi"() -> (w1164:refnum<vi>)
                n227 = invoke class="VI" method="FP.Open"(reference=w1164, error in=w1160) -> (reference out=w1163:refnum<vi>, error out=w1161:errorcluster)  [unwired: 3 in, 3 out]
                n228 = Close Reference(reference=w1163, error in (no error)=w1161) -> (error out=w1162:errorcluster)
              }
              frame "Write to VISA instrument" {
                n229 = call "WriteVISA_popup.vi"("error in (no error)"=w1165) -> ("Output Line Command"=w1166:string, "Cancel"=w1169:bool, "error out"=w1168:errorcluster)  [unwired: 8 in]
              }
            }
            n230 = local read "error\ncheck"() -> (w1041:bool)
            n231 = case shown="True" w1041 {
              tunnel: w1045 -> [_ w1062]
              tunnel: [FALSE ("error") w1060] -> w1044
              tunnel: w1040 -> [_ w1059]
              tunnel: w1039 -> [_ w1058]
              tunnel: w1038 -> [_ w1057]
              frame False {
              }
              frame True {
                n232 = Build Array(w1062) -> (w1061:string[])
                n233 = call "sequence util_error check.vi"("Sequences folder path"=w1057, "Use absolute sequence path"=w1059, "platform"=w1058, "Item Names IN"=w1061) -> ("error"=w1060:bool)  [unwired: 5 in, 1 out]
              }
            }
            n234 = Or(x=w1043, y=w1044) -> (x .or. y?=w1042:bool)
            n235 = Bundle By Name(cluster=w1048, "Signal"=w1043, "Command"=w1045, "Add or modification"=w1047) -> (w1046:T3)
            n236 = case shown="False" w1042 {
              tunnel: w1049 -> [w1065 _]
              tunnel: w1046 -> [w1064 _]
              tunnel: [w1063 w1066] -> w1050
              tunnel: w1051 -> [_ w1066]
              frame False {
                n237 = Generate User Event(user event=w1065, event data cluster=w1064) -> (error out=w1063:errorcluster)  [unwired: 2 in, 1 out]
              }
              frame True {
              }
            }
          }
          event "Sequence": Double Click {
            # "check if the sequence is changed. Returns 'False\"\nIf (1) 'cancel' button pressed \nOR (2) 'ok' button pressed but no value change"
            n238 = event-data() -> ("Row"=w1171:i32)  [unwired: 1 in]
            "Row" <- w1171
            n239 = Bundle By Name(cluster=w1198, "No. of line"=w1171) -> (w1197:T4)
            n240 = Unbundle By Name(w1189) -> ("Sequence Reference"=w1193:refnum<vi>)
            n241 = call "Library2.vi"("Message_command_in"=w1197, "error in (no error)"=w1196) -> ("Message_command out"=w1195:T5, "error out"=w1192:errorcluster)  [unwired: 7 in]
            n242 = property class="LstBox (strict)"(reference=w1193, error in=w1192) -> (error out=w1191:errorcluster, "Item Names"=w1190:string[])  [unwired: 1 out]
            n243 = Unbundle By Name(w1195) -> ("No. of command"=w1194:i32)
            n244 = local read "error\ncheck"() -> (w1175:bool)
            n245 = Index Array(array=w1190, index=w1171) -> (element=w1180:string)
            n246 = case shown="0" w1194 {
              tunnel: w1191 -> [w1221 w1228 w1235 w1242 w1249 w1258 w1267 w1274 w1281 w1288 w1295 w1302 w1303 w1316 w1320]
              tunnel: w1180 -> [w1220 w1227 w1234 w1241 w1248 w1253 w1266 w1273 w1280 w1287 w1294 w1301 w1307 w1315 _]
              tunnel: w1189 -> [w1218 w1225 w1232 w1239 w1246 w1260 w1264 w1271 w1278 w1285 w1292 w1299 w1309 w1313 w1319]
              tunnel: w1188 -> [w1217 w1224 w1231 w1238 w1245 w1259 w1263 w1270 w1277 w1284 w1291 w1298 w1308 w1312 w1318]
              tunnel: [w1219 w1226 w1233 w1240 w1247 w1255 w1265 w1272 w1279 w1286 w1293 w1296 w1306 w1314 w1320] -> w1185
              tunnel: [w1218 w1225 w1232 w1239 w1246 w1260 w1264 w1271 w1278 w1285 w1292 w1299 w1309 w1313 w1319] -> w1187
              tunnel: [w1217 w1224 w1231 w1238 w1245 w1259 w1263 w1270 w1277 w1284 w1291 w1298 w1308 w1312 w1318] -> w1186
              tunnel: [w1216 w1223 w1230 w1237 w1244 w1256 w1262 w1269 w1276 w1282 w1289 w1297 w1305 w1311 TRUE ("Cancel")] -> w1181
              tunnel: [w1215 w1222 w1229 w1236 w1243 w1257 w1261 w1268 w1275 w1283 w1290 w1300 w1304 w1310 _] -> w1178
              tunnel: w1172 -> [_ _ _ _ _ w1252 _ _ _ _ _ _ _ _ _]
              tunnel: w1174 -> [_ _ _ _ _ w1251 _ _ _ _ _ _ _ _ _]
              tunnel: w1173 -> [_ _ _ _ _ w1250 _ _ _ _ _ _ _ _ _]
              frame 0 {
                n247 = call "SetField_popup.vi"("error in (no error)"=w1221, "Input Line command"=w1220) -> ("Output Line command"=w1215:string, "Cancel"=w1216:bool, "error out"=w1219:errorcluster)  [unwired: 4 in]
              }
              frame 1 {
                n248 = call "SetTemp_popup.vi"("Input Line Command"=w1227, "error in (no error)"=w1228) -> ("error out"=w1226:errorcluster, "Cancel"=w1223:bool, "Output Line Command"=w1222:string)  [unwired: 6 in]
              }
              frame 2 {
                n249 = call "SetStart_popup.vi"("Input Line Command"=w1234, "error in (no error)"=w1235) -> ("Output Line Command"=w1229:string, "Cancel"=w1230:bool, "error out"=w1233:errorcluster)  [unwired: 6 in]
              }
              frame 4 {
                n250 = call "SetWaitForTemp_popup.vi"("Input Line Command"=w1241, "error in (no error)"=w1242) -> ("Output Line Command"=w1236:string, "Cancel"=w1237:bool, "error out"=w1240:errorcluster)  [unwired: 6 in]
              }
              frame 7 {
                n251 = call "SetRemarks_popup.vi"("Input Line Command"=w1248, "error in (no error)"=w1249) -> ("Cancel"=w1244:bool, "Output Line Command"=w1243:string, "error out"=w1247:errorcluster)  [unwired: 6 in]
              }
              frame 8 {
                n252 = call "RunMacro_popup.vi"("load?"=TRUE, "platform"=w1252, "command in"=w1253, "error in (no error)"=w1258, "abs. path"=w1251, "sequence folder"=w1250) -> ("Cancel"=w1256:bool, "command out"=w1257:string, "error out"=w1255:errorcluster)  [unwired: 2 in]
              }
              frame 9 {
                n253 = call "SetRunVI_popup.vi"("Input Line Command"=w1266, "error in (no error)"=w1267) -> ("Cancel"=w1262:bool, "Output Line Command"=w1261:string, "error out"=w1265:errorcluster)  [unwired: 6 in]
              }
              frame 10 {
                n254 = call "SetAbortVI_popup.vi"("Input Line Command"=w1273, "error in (no error)"=w1274) -> ("Cancel"=w1269:bool, "Output Line Command"=w1268:string, "error out"=w1272:errorcluster)  [unwired: 6 in]
              }
              frame 11 {
                n255 = call "SetDevice_popup.vi"("Input Line Command"=w1280, "error in (no error)"=w1281) -> ("Cancel"=w1276:bool, "Output Line Command"=w1275:string, "error out"=w1279:errorcluster)  [unwired: 6 in]
              }
              frame 12 {
                n256 = call "SetWaitFor_popup.vi"("Input Line Command"=w1287, "error in (no error)"=w1288) -> ("error out"=w1286:errorcluster, "Cancel"=w1282:bool, "Output Line Command"=w1283:string)  [unwired: 6 in]
              }
              frame 13 {
                n257 = call "SetParameter_popup.vi"("Input Line Command"=w1294, "error in (no error)"=w1295) -> ("error out"=w1293:errorcluster, "Cancel"=w1289:bool, "Output Line Command"=w1290:string)  [unwired: 6 in]
              }
              frame 14 {
                n258 = call "SetWaitForAnyVI_popup.vi"("Input Line Command"=w1301, "error in (no error)"=w1302) -> ("error out"=w1296:errorcluster, "Cancel"=w1297:bool, "Output Line Command"=w1300:string)  [unwired: 6 in]
              }
              frame 15 {
                n259 = call "WriteVISA_popup.vi"("error in (no error)"=w1303, "Input Line Command"=w1307) -> ("Output Line Command"=w1304:string, "Cancel"=w1305:bool, "error out"=w1306:errorcluster)  [unwired: 7 in]
              }
              frame 16 {
                n260 = call "SetSweep_popup.vi"("Input Line Command"=w1315, "error in (no error)"=w1316) -> ("Cancel"=w1311:bool, "Output Line Command"=w1310:string, "error out"=w1314:errorcluster)  [unwired: 6 in]
              }
              frame Default {
              }
            }
            n261 = case shown="True" w1175 {
              tunnel: w1178 -> [_ w1205]
              tunnel: [FALSE ("error") w1203] -> w1179
              tunnel: w1172 -> [_ w1202]
              tunnel: w1174 -> [_ w1201]
              tunnel: w1173 -> [_ w1200]
              frame False {
              }
              frame True {
                n262 = Build Array(w1205) -> (w1204:string[])
                n263 = call "sequence util_error check.vi"("Sequences folder path"=w1200, "Use absolute sequence path"=w1201, "platform"=w1202, "Item Names IN"=w1204) -> ("error"=w1203:bool)  [unwired: 5 in, 1 out]
              }
            }
            n264 = Equal?(x=w1180, y=w1178) -> (x = y?=w1182:bool)
            n265 = Or(x=w1181, y=w1182) -> (x .or. y?=w1177:bool)
            n266 = Or(x=w1177, y=w1179) -> (x .or. y?=w1176:bool)
            n267 = case shown="False" w1176 {
              selector: w1176 -> [w1208 _]
              tunnel: w1187 -> [w1212 _]
              tunnel: w1186 -> [w1210 _]
              tunnel: w1178 -> [w1209 _]
              tunnel: w1185 -> [w1207 w1214]
              tunnel: [w1206 w1214] -> w1184
              frame False {
                n268 = Bundle By Name(cluster=w1212, "Signal"=w1208, "Command"=w1209, "Add or modification"=FALSE) -> (w1211:T3)
                n269 = Generate User Event(user event=w1210, event data cluster=w1211, error in=w1207) -> (error out=w1206:errorcluster)  [unwired: 1 in, 1 out]
              }
              frame True {
              }
            }
          }
          event "horizontal lines", "line numbers": Value Change {
            w1323 = -208
            w1322 = 604
            n270 = event-data() -> ()  [unwired: 1 in, 6 out]
            n271 = case shown="True" "line numbers" {
              tunnel: [24 60] -> w1327
              tunnel: [840 804] -> w1328
              frame False {
              }
              frame True {
              }
            }
            n272 = property on="Sequence" class="LstBox (strict)"("Horizontal Lines Visible"="horizontal lines", "Left"=w1327, "Top"=w1323, "Height"=w1322, "Width"=w1328) -> ()  [unwired: 2 in, 2 out]
            n273 = property on="index" class="LstBox (strict)"("Horizontal Lines Visible"="horizontal lines", "Visible"="line numbers", "Left"=26, "Top"=w1323, "Height"=w1322, "Width"=41) -> ()  [unwired: 2 in, 2 out]
          }
          event "Sequence": Value Change; "Sequence": Mouse Wheel {
            n274 = event-data() -> ()  [unwired: 1 in, 4 out]
            n275 = local read "Sequence"() -> (w1334:i32[])
            n276 = Index Array(array=w1334, index=0) -> (element=w1333:i32)
            "Cursor Position" <- w1333
            n277 = property on="Sequence" class="LstBox (strict)"() -> ("Top Row"=w1335:i32)  [unwired: 2 in, 2 out]
            n278 = Replace Array Subset(array=w1334, new element=w1333, index=0) -> (w1336:i32[])
            n279 = local write "index"(w1336) -> ()
            n280 = property on="index" class="LstBox (strict)"("Top Row"=w1335) -> ()  [unwired: 2 in, 2 out]
          }
          event "Pause Button": Value Change {
            # "Note: unpause restart the execution line. For example, if it was paused\nduring 'Wait for 1 hr' line, the stopwatch will reset after unpause (waiting\nanother 1 hr). \nFor the subsequence, it restarts the line of the subsequence."
            # "for the looped command, \npause will stop the loop,\nunpause will resume the loop"
            n281 = event-data() -> ("NewVal"=w1345:bool)  [unwired: 1 in]
            n282 = local read "Current Line"() -> (w1344:i32)
            n283 = case shown="True" w1345 {
              tunnel: w1348 -> [w1355 w1365]
              tunnel: w1347 -> [_ w1364]
              tunnel: w1346 -> [w1351 w1363]
              tunnel: w1345 -> [_ w1361]
              tunnel: w1344 -> [w1354 w1360]
              tunnel: [w1353 w1357] -> w1343
              tunnel: [FALSE ("loop stop") TRUE ("loop stop")] -> w1341
              frame False {
                n284 = Decrement(x=w1354) -> (x-1=w1352:i32)
                n285 = Bundle By Name(cluster=w1351, "No. of line"=w1352) -> (w1350:T4)
                n286 = call "go_to_next_line.vi"("Message_command in"=w1350, "Command Queue in"=w1355) -> ("error out"=w1353:errorcluster)  [unwired: 8 in, 1 out]
              }
              frame True {
                n287 = flat-sequence {
                  frame #0 {
                    w1368 = "RunMacro.vi" ("VI Name")
                    n288 = local read "macro line"() -> (w1366:i32)
                    n289 = call "set_control_in_Memory.vi"("Control Name"="restart line", "Value"=w1366, "VI Name"=w1368) -> ()  [unwired: 2 in, 1 out]
                    n290 = call "set_control_in_Memory.vi"("Control Name"="paused?", "Value"=TRUE ("loop stop"), "VI Name"=w1368) -> ()  [unwired: 2 in, 1 out]
                  }
                }
                n291 = Bundle By Name(cluster=w1363, "No. of command"=1002, "Boolean"=w1361, "No. of line"=w1360, "Status"="Pause" ("Sequence status")) -> (w1359:T4)
                n292 = Enqueue Element At Opposite End(queue=w1365, element=w1359, error in (no error)=w1364) -> (error out=w1357:errorcluster)  [unwired: 1 in, 2 out]
              }
            }
          }
          event User Event; "reset\ncursor": Value Change {
            # "cursor\nreset button\npressed"
            n293 = event-data() -> ("Source"=w1374:T6)  [unwired: 1 in, 2 out]
            n294 = local read "track \nseq."() -> (w1372:bool)
            n295 = Equal To 0?(x=w1374) -> (x = 0?=w1373:bool)
            n296 = Or(x=w1373, y=w1372) -> (x .or. y?=w1371:bool)
            n297 = case shown="True" w1371 {
              frame False {
              }
              frame True {
                w1383 = 10  # halfline
                n298 = local read "Current Line"() -> (w1378:i32)
                n299 = local read "Sequence"() -> (w1382:i32[])
                n300 = Subtract(x=w1378, y=w1383) -> (x-y=w1379:i32)
                n301 = Replace Array Subset(array=w1382, new element=w1378, index=0) -> (w1377:i32[])
                n302 = Max & Min(x=u8 0, y=w1379) -> (max(x,y)=w1376:i32)  [unwired: 1 out]
                n303 = local write "Cursor Position"(w1378) -> ()
                n304 = local write "Sequence"(w1377) -> ()
                n305 = property on="Sequence" class="LstBox (strict)"("Top Row"=w1376) -> ()  [unwired: 2 in, 2 out]
                n306 = property on="index" class="LstBox (strict)"("Top Row"=w1376) -> ()  [unwired: 2 in, 2 out]
                n307 = local write "index"(w1377) -> ()
              }
            }
          }
          event "Skip Button": Value Change {
            n308 = event-data() -> ()  [unwired: 1 in, 1 out]
            n309 = Bundle By Name(cluster=w1393, "No. of command"=1004) -> (w1390:T4)
            n310 = Flush Queue(queue=w1389, error in (no error)=w1387) -> (queue out=w1388:refnum<queue>, error out=w1386:errorcluster)  [unwired: 1 out]
            n311 = Enqueue Element At Opposite End(queue=w1388, element=w1390, error in (no error)=w1386) -> (error out=w1392:errorcluster)  [unwired: 1 in, 2 out]
          }
          event "Sequence_Stop": Value Change {
            n312 = event-data() -> ("NewVal"=w1401:bool)  [unwired: 1 in]
            n313 = local read "Current Line"() -> (w1400:i32)
            n314 = Bundle By Name(cluster=w1402, "No. of command"=1003, "Boolean"=w1401, "No. of line"=w1400, "Status"="Pause" ("Sequence status")) -> (w1397:T4)
            n315 = Enqueue Element At Opposite End(queue=w1404, element=w1397, error in (no error)=w1403) -> (error out=w1399:errorcluster)  [unwired: 1 in, 2 out]
          }
          event "Program Stop": Value Change {
            n316 = event-data() -> ("NewVal"=w1410:bool)  [unwired: 1 in]
            n317 = Bundle By Name(cluster=w1409, "No. of command"=1005) -> (w1407:T4)
            n318 = Enqueue Element At Opposite End(queue=w1405, element=w1407, error in (no error)=w1406) -> (error out=w1411:errorcluster)  [unwired: 1 in, 2 out]
          }
          event "help": Value Change {
            n319 = event-data() -> ()  [unwired: 1 in, 1 out]
            n320 = Bundle By Name(cluster=w1417, "No. of command"=1006) -> (w1415:T4)
            n321 = Enqueue Element At Opposite End(queue=w1413, element=w1415, error in (no error)=w1414) -> (error out=w1418:errorcluster)  [unwired: 1 in, 2 out]
          }
          event Application Instance Close? {
            n322 = event-data() -> ()  [unwired: 1 in, 5 out]
            n323 = event-data("SilentShutdown"=TRUE) -> ()  [unwired: 1 in, 1 out]
          }
          event "sequence utility": Value Change {
            # "If true, current sequence and file path will be exported."
            n324 = event-data() -> ("CtlRef"=w1430:refnum<vi>)  [unwired: 1 in, 5 out]
            n325 = property on="Sequence" class="LstBox (strict)"() -> ("Item Names"=w1424:string[])  [unwired: 2 in, 2 out]
            n326 = property class="Bool (strict)"(reference=w1430, error in=w1429, "Value"=FALSE) -> (error out=w1428:errorcluster)  [unwired: 1 out]
            n327 = local read "Path"() -> (w1425:path)
            n328 = call "sequence utility.vi"("sequence in"=w1424, "error in (no error)"=w1428, "sequence path"=w1425, "platform"=w1432, "export?"=TRUE) -> ("error out"=w1427:errorcluster, "changed sequence"=w1422:string[], "do not update seq."=w1423:bool)  [unwired: 4 in]
            n329 = case shown="False" w1423 {
              tunnel: w1422 -> [w1433 _]
              frame False {
                n330 = property on="Sequence" class="LstBox (strict)"("Item Names"=w1433) -> ()  [unwired: 2 in, 2 out]
              }
              frame True {
              }
            }
          }
          event "exec window": Value Change {
            n331 = event-data() -> ("CtlRef"=w1448:refnum<vi>)  [unwired: 1 in, 5 out]
            n332 = Current VI's Path() -> (path=w1434:path)
            n333 = case shown="1" w1437 {
              tunnel: ["Monovu subvis/MonoVu_exec window.vi" ("name or relative path") "Monovu subvis\\MonoVu_exec window.vi" ("name or relative path")] -> w1444
              frame 0, Default {
              }
              frame 1 {
              }
            }
            n334 = flat-sequence {
              tunnel: [w1451] -> w1435
              tunnel: w1434 -> [w1451]
              frame #0 {
                (unwired) string[] [] ("sequence contents")
                n335 = property on="Sequence" class="LstBox (strict)"() -> ("Item Names"=→"sequence contents":string[])  [unwired: 2 in, 2 out]
              }
            }
            n336 = property class="Bool (strict)"(reference=w1448, error in=w1447, "Value"=FALSE) -> (error out=w1446:errorcluster)  [unwired: 1 out]
            n337 = Strip Path(path=w1435) -> (stripped path=w1441:path)  [unwired: 1 out]
            n338 = Build Path(base path=w1441, name or relative path=w1444) -> (appended path=w1436:path)
            n339 = Open VI Reference(vi path=w1436) -> (vi reference=w1443:refnum<vi>, error out=w1442:errorcluster)  [unwired: 5 in]
            n340 = invoke class="VI" method="FP.Open"(reference=w1443, error in=w1442) -> (reference out=w1440:refnum<vi>)  [unwired: 3 in, 4 out]
            n341 = invoke class="VI" method="Run VI"(reference=w1440, "Wait until done"=FALSE ("Wait Until Done")) -> (reference out=w1438:refnum<vi>)  [unwired: 3 in, 4 out]
            n342 = Close Reference(reference=w1438) -> ()  [unwired: 1 in, 1 out]
          }
        }
        n343 = local write "loop stop"(w530) -> ()
      }
      n344 = while {
        shift-right: [w98] -> _
        shift-left: w57 -> [w99]
        tunnel: w52 -> [w97]
        tunnel: w56 -> [w96]
        tunnel: w55 -> [w95]
        tunnel: [w78] -> w49
        tunnel: w54 -> [w89]
        tunnel: w53 -> [w93]
        tunnel: "PS Control VI Name" -> [w71]
        tunnel: w46 -> [w70]
        tunnel: w45 -> [w62]
        tunnel: w43 -> [w64]
        i -> [w85]
        stop <- w104 stop-if-true
        # "Message_Handler"
        n345 = Dequeue Element(queue=w97, error in (no error)=w96) -> (queue out=w102:refnum<queue>, element=w101:T4, error out=w103:errorcluster)  [unwired: 1 in, 1 out]
        n346 = Unbundle By Name(w101) -> ("No. of command"=w100:i32, "Subsequence"=w88:string[], "No. of line"=w63:i32)
        "macro line" <- w63
        n347 = Array Size(array=w88) -> (size(s)=w90:i32)
        n348 = case shown="1" w90 {
          tunnel: w88 -> [_ w117]
          tunnel: [w108 w113] -> w72
          tunnel: [w109 w110] -> w86
          tunnel: w63 -> [w109 w112]
          tunnel: [w108 w111] -> w74
          frame 0, Default {
            (unwired) FALSE ("Visible")
            w108 = ""
          }
          frame 1 {
            (unwired) TRUE ("Visible")
            n349 = Number To Decimal String(number=w112) -> (decimal integer string=w114:string)  [unwired: 1 in]
            n350 = local read "macro cmd no"() -> (w110:i32)
            n351 = Index Array(array=w117, index=0) -> (element=w111:string)
            n352 = Concatenate Strings(w111, w114, "\n") -> (w113:string)
          }
        }
        n353 = case shown="1006" w100 {
          tunnel: [_ _ _ _ _ _ _ _ _ _ _ _ _ _ _ _ FALSE _ _ _ _ TRUE _ _ _] -> w104
          tunnel: w103 -> [w125 w140 w153 w165 w177 w190 w206 w225 w237 w249 w260 w270 w284 w308 w346 w357 w369 w397 w431 w446 w469 w476 _ w505 w526]
          tunnel: [w119 w131 w143 w156 w168 w181 w193 w218 w228 w240 w253 w265 w275 w295 w336 w350 w367 w387 w427 w437 w450 w476 _ w496 w519] -> w94
          tunnel: w101 -> [w130 w134 w149 w161 w172 w187 w204 w215 w235 w247 w261 w273 w282 w291 w342 w358 _ _ _ _ w456 _ _ _ w523]
          tunnel: w102 -> [w129 w137 w150 w162 w176 w188 w207 w223 w234 w246 w262 w274 w285 w296 w343 w359 _ w395 w432 w447 w470 _ _ w516 w524]
          tunnel: w99 -> [w126 w141 w154 w166 w179 w191 w208 w226 w239 w251 w264 w268 w287 w310 w348 w361 w379 w390 w436 w444 w473 w477 w488 w506 w527]
          tunnel: [w123 w138 w152 w164 w178 w189 w205 w224 w238 w250 w263 w267 w286 w309 w347 w360 w371 w389 w435 w445 w472 w477 w488 w507 w525] -> w98
          tunnel: w95 -> [_ _ _ _ _ _ _ _ _ _ _ _ _ _ _ _ _ _ _ _ _ _ _ _ _]
          tunnel: w89 -> [_ _ _ _ _ _ _ _ _ _ _ _ _ _ _ _ _ _ _ _ _ _ _ _ _]
          tunnel: w93 -> [_ _ _ _ _ _ _ _ _ _ _ _ _ _ _ _ _ w383 _ _ _ _ _ w502 _]
          tunnel: [w120 w132 w145 w157 w169 w182 w195 w220 w230 w242 w255 w266 w278 w288 w344 w352 w366 w388 w433 w448 w464 0 ("No. of line") w486 w491 w521] -> w68
          tunnel: [w127 w142 w155 w167 w173 w184 w202 _ w231 w243 w257 w271 w279 _ w345 w354 "Idle" ("Status") "Idle or Waiting for the command complete" ("Status") "Pause" ("Status") "Idle" ("Status") "Skip" ("Sequence status") "Program Close" ("Sequence status") _ _ _] -> w91
          tunnel: FALSE ("Use LS336Panel.vi") -> [_ w133 _ _ w170 _ _ _ _ _ _ _ _ _ _ _ _ _ _ _ _ _ _ _ _]
          tunnel: "Magnet PS" -> [w121 _ _ _ _ w183 _ _ _ _ _ _ _ _ _ _ _ _ _ _ _ _ _ _ _]
          tunnel: w86 -> [w120 w132 w145 w157 w169 w182 w195 w220 w230 w242 w255 w266 w278 w288 w344 w352 _ _ _ _ _ _ w486 w491 w521]
          tunnel: [w119 w131 w143 w156 w168 w181 w192 w218 w227 _ w252 w265 w277 w295 w338 w349 w367 w384 w427 w437 w450 w476 errorcluster {"status"=FALSE, "code"=0, "source"=""} ("error out") w495 w519] -> w76
          tunnel: w74 -> [_ _ _ _ _ _ _ _ _ _ _ _ _ _ _ _ _ _ _ _ _ _ _ w494 _]
          tunnel: w72 -> [_ _ _ _ _ _ _ _ _ _ _ _ _ w294 _ _ _ _ _ _ _ _ _ _ _]
          tunnel: w71 -> [w118 _ _ _ _ w180 _ _ _ _ _ _ _ _ _ _ _ _ _ _ _ _ _ _ _]
          tunnel: w70 -> [_ _ _ _ _ _ _ _ _ _ _ _ _ _ _ _ _ _ _ _ _ _ _ _ _]
          tunnel: "Use absolute sequence path" -> [_ _ _ _ _ _ _ w211 _ _ _ _ _ _ _ _ _ _ _ _ _ _ _ _ _]
          tunnel: "Sequences folder path" -> [_ _ _ _ _ _ _ w210 _ _ _ _ _ _ _ _ _ _ _ _ _ _ _ _ _]
          tunnel: w64 -> [_ _ _ _ _ _ _ w209 _ _ _ _ _ _ _ _ _ _ _ _ _ _ w485 _ _]
          tunnel: w63 -> [_ _ _ _ _ _ _ _ _ _ _ _ _ _ _ _ w366 _ _ _ _ _ _ _ _]
          tunnel: w62 -> [_ _ _ _ _ _ _ _ _ _ _ _ _ w289 _ _ _ _ _ _ _ _ _ _ _]
          frame 0 {
            # "Set Field"
            n354 = call "Start_Initial.vi"("error in (no error)"=w125, "Reference"=w126) -> ("error out"=w124:errorcluster, "dup Reference"=w123:T7)  [unwired: 8 in]
            n355 = call "Set_Field.vi"("Magnet PS"=w121, "error in (no error)"=w124, "PS Control VI Name"=w118, "Command_message_in"=w130, "Command_queue_in"=w129) -> ("error out"=w119:errorcluster, "Command_message_out"=w128:T5)  [unwired: 4 in, 1 out]
            n356 = Wait (ms)(milliseconds to wait=u32 100) -> ()  [unwired: 1 out]
            n357 = Unbundle By Name(w128) -> ("Status"=w127:string)
          }
          frame 1 {
            # "Set Temp"
            n358 = call "Start_Initial.vi"("error in (no error)"=w140, "Reference"=w141) -> ("error out"=w139:errorcluster, "dup Reference"=w138:T7)  [unwired: 8 in]
            n359 = call "Set_Temp.vi"("LS336FrontPanel.vi"=w133, "error in (no error)"=w139, "Message_command_in"=w134, "Command_queue_in"=w137) -> ("error out"=w131:errorcluster, "Message_command_out"=w136:T5)  [unwired: 6 in]
            n360 = Wait (ms)(milliseconds to wait=u32 100) -> ()  [unwired: 1 out]
            n361 = Unbundle By Name(w136) -> ("Status"=w142:string)
          }
          frame 2 {
            # "Start DAQ"
            n362 = control-ref of="NML Data Acquisition VI"() -> (w147:refnum<vi>)
            n363 = call "Start_Initial.vi"("error in (no error)"=w153, "Reference"=w154) -> ("error out"=w151:errorcluster, "dup Reference"=w152:T7)  [unwired: 8 in]
            n364 = local read "platform"() -> (w144:u16)
            n365 = call "Start_DAQ.vi"("platform"=w144, "error in (no error)"=w151, "Command_Queue_in"=w150, "Command_message_in"=w149, "DAQ in"=w147) -> ("error out"=w143:errorcluster, "Command_message_out"=w148:T5)  [unwired: 5 in]
            n366 = Unbundle By Name(w148) -> ("Status"=w155:string)
            n367 = Wait (ms)(milliseconds to wait=u32 100) -> ()  [unwired: 1 out]
          }
          frame 3 {
            # "Stop DAQ"
            n368 = control-ref of="NML Data Acquisition VI"() -> (w159:refnum<vi>)
            n369 = call "Start_Initial.vi"("error in (no error)"=w165, "Reference"=w166) -> ("error out"=w163:errorcluster, "dup Reference"=w164:T7)  [unwired: 8 in]
            n370 = call "Stop_DAQ.vi"("error in (no error)"=w163, "Command_Queue_in"=w162, "Command_message_in"=w161, "DAQ in"=w159) -> ("error out"=w156:errorcluster, "Command_message_out"=w160:T5)  [unwired: 6 in]
            n371 = Unbundle By Name(w160) -> ("Status"=w167:string)
            n372 = Wait (ms)(milliseconds to wait=u32 100) -> ()  [unwired: 1 out]
          }
          frame 4 {
            # "Wait for Temperature"
            n373 = call "Start_Initial.vi"("error in (no error)"=w177, "Reference"=w179) -> ("error out"=w175:errorcluster, "dup Reference"=w178:T7)  [unwired: 8 in]
            n374 = Wait (ms)(milliseconds to wait=u32 100) -> ()  [unwired: 1 out]
            n375 = call "Wait_for_Temp.vi"("LS336FrontPanel.vi"=w170, "error in (no error)"=w175, "Message_command in"=w172, "Command Queue"=w176) -> ("error out"=w168:errorcluster, "dup Message_command"=w174:T5)  [unwired: 6 in]
            n376 = Unbundle By Name(w174) -> ("Status"=w173:string)
          }
          frame 5 {
            # "Wait for Field Stable"
            n377 = call "Start_Initial.vi"("error in (no error)"=w190, "Reference"=w191) -> ("error out"=w186:errorcluster, "dup Reference"=w189:T7)  [unwired: 8 in]
            n378 = call "Wait_for_field_stable.vi"("Magnet PS"=w183, "error in (no error)"=w186, "PS Control VI Name"=w180, "Message_command in"=w187, "Command_Queue"=w188) -> ("error out"=w181:errorcluster, "Message_command out"=w185:T5)  [unwired: 5 in]
            n379 = Unbundle By Name(w185) -> ("Status"=w184:string)
          }
          frame 7 {
            # "Remarks"
            n380 = call "Start_Initial.vi"("error in (no error)"=w206, "Reference"=w208) -> ("error out"=w203:errorcluster, "dup Reference"=w205:T7)  [unwired: 8 in]
            n381 = call "Library2.vi"("Message_command_in"=w204, "error in (no error)"=w203) -> ("Message_command out"=w197:T5, "error out"=w194:errorcluster)  [unwired: 7 in]
            n382 = Unbundle By Name(w197) -> ("Sequence_History"=w201:string, "Status"=w200:string)
            n383 = Concatenate Strings(w201, w200, "\r") -> (w198:string)
            n384 = Bundle By Name(cluster=w197, "Sequence_History"=w198) -> (w196:T5)
            n385 = call "go_to_next_line.vi"("error in (no error)"=w194, "Message_command in"=w196, "Command Queue in"=w207) -> ("error out"=w193:errorcluster)  [unwired: 7 in, 1 out]
            n386 = Unbundle By Name(w197) -> ("Status"=w202:string)
            n387 = Merge Errors(w194, w193) -> (w192:errorcluster)
          }
          frame 8 {
            # "Run Macro"
            n388 = call "Start_Initial.vi"("error in (no error)"=w225, "Reference"=w226) -> ("error out"=w222:errorcluster, "dup Reference"=w224:T7)  [unwired: 8 in]
            n389 = Unbundle By Name(w215) -> ("Status"=w214:string)
            n390 = Unbundle By Name(w215) -> ("No. of line"=w221:i32)
            n391 = Match Pattern(string=w214, regular expression="Run Macro ") -> (after substring=w212:string)  [unwired: 1 in, 3 out]
            n392 = Concatenate Strings("Macro Started: " ("input"), w212) -> (w216:string)
            n393 = property on="macro cmd no" class="DigNum (strict)"("Value"=w221) -> ()  [unwired: 2 in, 2 out]
            n394 = call "RunMacro.vi"("abs. path"=w211, "sequence folder"=w210, "submacro"=FALSE, "error in (no error)"=w222, "platform"=w209, "Message_command"=w215, "queue"=w223) -> ("error out"=w218:errorcluster)  [unwired: 2 in, 2 out]
            n395 = call "write to log file.vi"("input"=w216) -> ()  [unwired: 9 in, 1 out]
          }
          frame 9 {
            # "Run VI"
            n396 = call "Start_Initial.vi"("error in (no error)"=w237, "Reference"=w239) -> ("error out"=w236:errorcluster, "dup Reference"=w238:T7)  [unwired: 8 in]
            n397 = call "Run_VI.vi"("error in (no error)"=w236, "Message_command_in"=w235, "Command Queue in"=w234) -> ("error out"=w229:errorcluster, "Message_command out"=w232:T5, "Command Queue out"=w233:T8)  [unwired: 5 in, 1 out]
            n398 = call "go_to_next_line.vi"("error in (no error)"=w229, "Message_command in"=w232, "Command Queue in"=w233) -> ("error out"=w228:errorcluster)  [unwired: 7 in, 1 out]
            n399 = Unbundle By Name(w232) -> ("Status"=w231:string)
            n400 = Merge Errors(w229, w228) -> (w227:errorcluster)
          }
          frame 10 {
            # "Error reporting disabled\nfor Abort.vi"
            # "Abort VI"
            n401 = call "Start_Initial.vi"("error in (no error)"=w249, "Reference"=w251) -> ("error out"=w248:errorcluster, "dup Reference"=w250:T7)  [unwired: 8 in]
            n402 = call "Abort_VI.vi"("error in (no error)"=w248, "Message_command_in"=w247, "Command Queue in"=w246) -> ("error out"=w241:errorcluster, "Message_command out"=w244:T5, "Command Queue out"=w245:T8)  [unwired: 5 in, 1 out]
            n403 = call "go_to_next_line.vi"("error in (no error)"=w241, "Message_command in"=w244, "Command Queue in"=w245) -> ("error out"=w240:errorcluster)  [unwired: 7 in, 1 out]
            n404 = Unbundle By Name(w244) -> ("Status"=w243:string)
          }
          frame 11 {
            # "Set Device"
            n405 = call "Start_Initial.vi"("error in (no error)"=w260, "Reference"=w264) -> ("error out"=w259:errorcluster, "dup Reference"=w263:T7)  [unwired: 8 in]
            n406 = call "Run_Device.vi"("error in (no error)"=w259, "Message_command"=w261, "Command Queue"=w262) -> ("error out"=w254:errorcluster, "dup Message_command"=w256:T5, "dup Command Queue"=w258:T8)  [unwired: 6 in]
            n407 = call "go_to_next_line.vi"("error in (no error)"=w254, "Message_command in"=w256, "Command Queue in"=w258) -> ("error out"=w253:errorcluster)  [unwired: 7 in, 1 out]
            n408 = Unbundle By Name(w256) -> ("Status"=w257:string)
            n409 = Merge Errors(w253, w254) -> (w252:errorcluster)
          }
          frame 12 {
            # "Wait for"
            n410 = call "Start_Initial.vi"("error in (no error)"=w270, "Reference"=w268) -> ("error out"=w269:errorcluster, "dup Reference"=w267:T7)  [unwired: 8 in]
            n411 = call "Wait_for.vi"("error in (no error)"=w269, "Message_command in"=w273, "Command Queue"=w274) -> ("error out"=w265:errorcluster, "dup Message_command"=w272:T5)  [unwired: 7 in]
            n412 = Unbundle By Name(w272) -> ("Status"=w271:string)
          }
          frame 13 {
            # "Set Parameter"
            n413 = call "Start_Initial.vi"("error in (no error)"=w284, "Reference"=w287) -> ("error out"=w283:errorcluster, "dup Reference"=w286:T7)  [unwired: 8 in]
            n414 = call "Set_Parameters.vi"("error in (no error)"=w283, "Message_command In"=w282, "Command Queue In"=w285) -> ("error out"=w276:errorcluster, "Message_command Out"=w280:T5, "Command Queue out"=w281:T8)  [unwired: 6 in]
            n415 = Unbundle By Name(w280) -> ("Status"=w279:string)
            n416 = call "go_to_next_line.vi"("error in (no error)"=w276, "Message_command in"=w280, "Command Queue in"=w281) -> ("error out"=w275:errorcluster)  [unwired: 7 in, 1 out]
            n417 = Merge Errors(w275, w276) -> (w277:errorcluster)
          }
          frame 14 {
            # "Wait for any VI value"
            n418 = call "Start_Initial.vi"("error in (no error)"=w308, "Reference"=w310) -> ("error out"=w307:errorcluster, "dup Reference"=w309:T7)  [unwired: 8 in]
            n419 = call "WaitForAnyVI_initialize.vi"("Message_command In"=w291) -> ("current time"=w299:timestamp, "parameters"=w301:string[], "vi reference"=w305:refnum<vi>, "application reference"=w306:refnum<vi>)  [unwired: 7 in]
            n420 = local write "loop stop"(FALSE ("loop stop")) -> ()
            n421 = while {
              shift-right: [w332] -> w298
              shift-left: w307 -> [w333]
              shift-right: [w331] -> w302
              shift-left: w306 -> [w328]
              shift-right: [w330] -> w303
              shift-left: w305 -> [w327]
              tunnel: w301 -> [w329]
              shift-right: [w324] -> _
              shift-left: u32 0 ("millisecond timer value") -> [w326]
              tunnel: w299 -> [w325]
              tunnel: w294 -> [w323]
              tunnel: [w321] -> w292
              tunnel: w289 -> [w316]
              tunnel: w288 -> [w311]
              stop <- w319 stop-if-true
              n422 = local read "Cursor Position"() -> (w315:i32)
              n423 = local read "track \nseq."() -> (w314:bool)
              n424 = local write "Current Line"(w311) -> ()
              n425 = Not Equal?(x=w311, y=w315) -> (x != y?=w313:bool)
              n426 = And(x=w313, y=w314) -> (x .and. y?=w312:bool)
              n427 = call "WaitForAnyVI.vi"("application reference"=w328, "vi reference"=w327, "Initial Time"=w325, "parameters"=w329, "error in (no error)"=w333, "counter in"=w326) -> ("counter out"=w324:i32, "status"=w321:string, "application reference out"=w331:refnum<vi>, "Done"=w318:bool, "vi reference out"=w330:refnum<vi>, "error out"=w332:errorcluster)  [unwired: 4 in]
              n428 = Concatenate Strings(w323, w321) -> (w322:string)
              n429 = case shown="True" w312 {
                tunnel: w316 -> [_ w334]
                frame False {
                }
                frame True {
                  n430 = Generate User Event(user event=w334, event data cluster=TRUE ("event data")) -> ()  [unwired: 2 in, 2 out]
                }
              }
              n431 = local write "Sequence Status"(w322) -> ()
              n432 = Or(x=w318, y="loop stop") -> (x .or. y?=w319:bool)
              n433 = Wait (ms)(milliseconds to wait="interval in a looped execution") -> ()  [unwired: 1 out]
            }
            n434 = Close Reference(reference=w303, error in (no error)=w298) -> (error out=w304:errorcluster)
            n435 = Bundle By Name(cluster=w291, "Status"=w292) -> (w293:T4)
            n436 = Close Reference(reference=w302, error in (no error)=w304) -> (error out=w297:errorcluster)
            n437 = call "go_to_next_line.vi"("error in (no error)"=w297, "Message_command in"=w293, "Command Queue in"=w296) -> ("error out"=w295:errorcluster)  [unwired: 7 in, 1 out]
          }
          frame 15 {
            # "Write to VISA"
            n438 = call "Start_Initial.vi"("error in (no error)"=w346, "Reference"=w348) -> ("error out"=w341:errorcluster, "dup Reference"=w347:T7)  [unwired: 8 in]
            n439 = call "Write2VISA.vi"("error in (no error)"=w341, "Message_command In"=w342, "Command Queue In"=w343) -> ("error out"=w337:errorcluster, "Message_command Out"=w339:T5, "Command Queue out"=w340:T8)  [unwired: 6 in]
            n440 = call "go_to_next_line.vi"("error in (no error)"=w337, "Message_command in"=w339, "Command Queue in"=w340) -> ("error out"=w336:errorcluster)  [unwired: 7 in, 1 out]
            n441 = Unbundle By Name(w339) -> ("Status"=w345:string)
            n442 = Merge Errors(w336, w337) -> (w338:errorcluster)
          }
          frame 16 {
            # "Sweep"
            n443 = call "Start_Initial.vi"("error in (no error)"=w357, "Reference"=w361) -> ("error out"=w356:errorcluster, "dup Reference"=w360:T7)  [unwired: 8 in]
            n444 = call "Sweep_device.vi"("error in (no error)"=w356, "Message_command"=w358, "Command Queue"=w359) -> ("error out"=w351:errorcluster, "dup Message_command"=w353:T5, "dup Command Queue"=w355:T8)  [unwired: 6 in]
            n445 = call "go_to_next_line.vi"("error in (no error)"=w351, "Message_command in"=w353, "Command Queue in"=w355) -> ("error out"=w350:errorcluster)  [unwired: 7 in, 1 out]
            n446 = Unbundle By Name(w353) -> ("Status"=w354:string)
            n447 = Merge Errors(w350, w351) -> (w349:errorcluster)
          }
          frame 1000, Default {
            # "Program Initialize"
            n448 = control-ref of="NML Data Acquisition VI"() -> (w373:refnum<vi>)
            n449 = control-ref of="Program Stop"() -> (w374:refnum<vi>)
            n450 = control-ref of="Sequence_Stop"() -> (w376:refnum<vi>)
            n451 = control-ref of="Sequence"() -> (w364:refnum<vi>)
            n452 = control-ref of="Run Sequence"() -> (w378:refnum<vi>)
            n453 = control-ref of="Pause Button"() -> (w377:refnum<vi>)
            n454 = control-ref of="Skip Button"() -> (w375:refnum<vi>)
            n455 = property class="LstBox (strict)"(reference=w364) -> ("Item Names"=w363:string[])  [unwired: 1 in, 2 out]
            n456 = Bundle By Name(cluster=w379, "Sequence_Run"=w378, "Sequence_Pause"=w377, "Sequence_Stop"=w376, "Sequence_Skip"=w375, "Program Stop"=w374, "Sequence"=w364, "NML Data Acquisition VI"=w373) -> (w372:T7)
            n457 = Array Size(array=w363) -> (size(s)=w362:i32)
            n458 = for {
              N: w362 -> [_]
              tunnel: [w380] -> w365 mode=indexing
              i -> [w381]
              n459 = Number To Decimal String(number=w381) -> (decimal integer string=w380:string)  [unwired: 1 in]
            }
            n460 = call "Program_initial.vi"("error in (no error)"=w369, "Reference"=w372) -> ("error out"=w367:errorcluster, "dup Reference"=w371:T7)  [unwired: 8 in]
            n461 = property on="index" class="LstBox (strict)"("Item Names"=w365) -> ()  [unwired: 2 in, 2 out]
          }
          frame 1001 {
            # "Run Sequence"
            n462 = Unbundle By Name(w390) -> ("Sequence"=w392:refnum<vi>)
            n463 = local read "error\ncheck"() -> (w382:bool)
            n464 = call "Sequence_Message_initial_line.vi"("reference"=w392, "error check?"=w382, "error in (no error)"=w397) -> ("Number of begin"=w393:u16, "Run?"=w396:bool, "error out"=w394:errorcluster)  [unwired: 5 in]
            n465 = case shown="True" w396 {
              tunnel: w395 -> [w408 w421]
              tunnel: w394 -> [w400 w413]
              tunnel: [w399 w409] -> w387
              tunnel: w383 -> [w401 w424]
              tunnel: w393 -> [w398 w414]
              tunnel: [w404 w420] -> _
              tunnel: w392 -> [_ w418]
              tunnel: w390 -> [w407 w417]
              tunnel: [w407 w415] -> w389
              tunnel: [w398 w414] -> w388
              tunnel: [w400 w410] -> w386
              tunnel: [w399 w409] -> w385
              frame False {
                n466 = Bundle By Name(cluster=w401, "No. of command"=1000, "No. of line"=w398) -> (w402:T4)
                n467 = Flush Queue(queue=w408, error in (no error)=w400) -> (queue out=w406:refnum<queue>, error out=w405:errorcluster)  [unwired: 1 out]
                n468 = Enqueue Element(queue=w406, element=w402, error in (no error)=w405) -> (queue out=w404:refnum<queue>, error out=w399:errorcluster)  [unwired: 1 in, 1 out]
              }
              frame True {
                n469 = Get Date/Time In Seconds() -> (seconds since 1Jan1904=w419:timestamp)
                n470 = Bundle By Name(cluster=w424, "No. of line"=w414, "Initial Time"=w419, "Sequence Ref."=w418) -> (w423:T4)
                n471 = call "Library2.vi"("Message_command_in"=w423, "error in (no error)"=w413) -> ("Message_command out"=w422:T5, "error out"=w410:errorcluster)  [unwired: 7 in]
                n472 = case shown="True" "override command error" {
                  tunnel: [w425 errorcluster {"status"=FALSE, "code"=0, "source"=""} ("error in (no error)")] -> w411
                  tunnel: w410 -> [w425 _]
                  frame False {
                  }
                  frame True {
                  }
                }
                n473 = Enqueue Element(queue=w421, element=w422, error in (no error)=w411) -> (queue out=w420:refnum<queue>, error out=w416:errorcluster)  [unwired: 1 in, 1 out]
                n474 = call "Start_Initial.vi"("error in (no error)"=w416, "Reference"=w417) -> ("error out"=w409:errorcluster, "dup Reference"=w415:T7)  [unwired: 8 in]
              }
            }
            n475 = Merge Errors(w386, w385) -> (w384:errorcluster)
          }
          frame 1002 {
            # "Sequence_Pause"
            n476 = Flush Queue(queue=w432, error in (no error)=w431) -> (error out=w430:errorcluster)  [unwired: 2 out]
            n477 = call "Pause_Initial.vi"("error in (no error)"=w430, "Blinking"=TRUE, "Reference"=w436) -> ("error out"=w427:errorcluster, "dup Reference"=w435:T7)  [unwired: 7 in]
            n478 = call "write to log file.vi"("input"="!!! Pause button pressed !!!") -> ()  [unwired: 9 in, 1 out]
            n479 = local read "Current Line"() -> (w433:i32)
          }
          frame 1003 {
            # "Sequence_Stop"
            n480 = local read "Current Line"() -> (w440:i32)
            n481 = Flush Queue(queue=w447, error in (no error)=w446) -> (error out=w443:errorcluster)  [unwired: 2 out]
            n482 = property on="Sequence" class="LstBox (strict)"() -> ("Item Names"=w439:string[])  [unwired: 2 in, 2 out]
            n483 = Index Array(array=w439, index=w440) -> (element=w441:string)
            n484 = Concatenate Strings("!!! Stop button pressed !!!" ("input"), w441) -> (w442:string)
            n485 = call "write to log file.vi"("input"=w442) -> ()  [unwired: 9 in, 1 out]
            n486 = local read "Current Line"() -> (w448:i32)
            n487 = call "Program_initial.vi"("error in (no error)"=w443, "Reference"=w444) -> ("error out"=w437:errorcluster, "dup Reference"=w445:T7)  [unwired: 8 in]
          }
          frame 1004 {
            # "1. skipped sequence is added in the log\n2. Checks if it is resulted from idle or not found command."
            # "Sequence_Skip"
            n488 = local read "Current Line"() -> (w458:i32)
            n489 = Get Date/Time In Seconds() -> (seconds since 1Jan1904=w466:timestamp)
            n490 = control-ref of="Sequence"() -> (w465:refnum<vi>)
            n491 = Flush Queue(queue=w470, error in (no error)=w469) -> (queue out=w468:refnum<queue>, error out=w467:errorcluster)  [unwired: 1 out]
            n492 = property on="Sequence" class="LstBox (strict)"() -> ("Item Names"=w459:string[])  [unwired: 2 in, 2 out]
            n493 = Bundle By Name(cluster=w456, "No. of line"=w458, "Initial Time"=w466, "Sequence Ref."=w465) -> (w463:T4)
            n494 = call "Start_Initial.vi"("error in (no error)"=w467, "Reference"=w473) -> ("error out"=w471:errorcluster, "dup Reference"=w472:T7)  [unwired: 8 in]
            n495 = Unbundle By Name(w456) -> ("Status"=w454:string)
            n496 = Index Array(array=w459, index=w458) -> (element=w457:string)
            n497 = Concatenate Strings("!!! SKIP !!! " ("string"), w457) -> (w451:string)
            n498 = Equal?(x=w454, y="Unidentified command. Skipped" ("Status")) -> (x = y?=w453:bool)
            n499 = case shown="True" w453 {
              tunnel: [w474 "doo nott write to log"] -> w452
              tunnel: w451 -> [w474 _]
              frame False {
              }
              frame True {
              }
            }
            n500 = Bundle By Name(cluster=w463, "Status"=w452) -> (w462:T4)
            n501 = Unbundle By Name(w462) -> ("No. of line"=w464:i32)
            n502 = call "go_to_next_line.vi"("error in (no error)"=w471, "Message_command in"=w462, "Command Queue in"=w468) -> ("error out"=w450:errorcluster)  [unwired: 7 in, 1 out]
          }
          frame 1005 {
            # "Program Stop"
          }
          frame 1006 {
            # "Open html help document"
            n503 = Current VI's Path() -> (path=w483:path)
            n504 = case shown="0, Default" w485 {
              tunnel: ["Monovu subvis/monovu help.html" ("string") "Monovu subvis\\monovu help.html" ("string")] -> w481
              frame 0, Default {
              }
              frame 1 {
              }
            }
            n505 = Strip Path(path=w483) -> (stripped path=w482:path)  [unwired: 1 out]
            n506 = Build Path(base path=w482, name or relative path=w481) -> (appended path=w484:path)
            n507 = call-poly <vilib>:"Open HTML Report in Browser.vi"("path"=w484) -> ()  [unwired: 13 in, 2 out]
          }
          frame 1007 {
            # "1. Delete queues of command lines in the subsequences\n2. Returns to the next line of the main sequences."
            # "END SUBsequence"
            n508 = Match Pattern(string=w494, regular expression=",  line #: " ("string")) -> (before substring=w492:string)  [unwired: 1 in, 3 out]
            n509 = Get Date/Time In Seconds() -> (seconds since 1Jan1904=w513:timestamp)
            n510 = Flush Queue(queue=w516, error in (no error)=w505) -> (queue out=w508:refnum<queue>, error out=w504:errorcluster)  [unwired: 1 out]
            n511 = Unbundle By Name(w506) -> ("Sequence"=w512:refnum<vi>)
            n512 = property on="macro cmd no" class="DigNum (strict)"() -> ("Value"=w515:i32)  [unwired: 2 in, 2 out]
            n513 = local read "override command error"() -> (w501:bool)
            n514 = Increment(x=w515) -> (x+1=w514:i32)
            n515 = Bundle By Name(cluster=w502, "No. of line"=w514, "Initial Time"=w513, "Sequence Ref."=w512, "Subsequence"=string[] []) -> (w511:T4)
            n516 = call "Library2.vi"("Message_command_in"=w511, "error in (no error)"=w504) -> ("Message_command out"=w509:T5, "error out"=w497:errorcluster)  [unwired: 7 in]
            n517 = case shown="True" w501 {
              tunnel: [w517 errorcluster {"status"=FALSE, "code"=0, "source"=""} ("error in (no error)")] -> w500
              tunnel: w497 -> [w517 _]
              frame False {
              }
              frame True {
              }
            }
            n518 = Concatenate Strings("Macro Ended: " ("input"), w492) -> (w498:string)
            n519 = Enqueue Element(queue=w508, element=w509, error in (no error)=w500) -> (error out=w510:errorcluster)  [unwired: 1 in, 2 out]
            n520 = call "write to log file.vi"("input"=w498) -> ()  [unwired: 9 in, 1 out]
            n521 = call "Start_Initial.vi"("error in (no error)"=w510, "Reference"=w506) -> ("error out"=w496:errorcluster, "dup Reference"=w507:T7)  [unwired: 8 in]
            n522 = Merge Errors(w497, w496) -> (w495:errorcluster)
          }
          frame 1008 {
            # "Nested submacros are unnested to make a single expanded macro (see\ncommand line 8)."
            # "SubMacro"
            n523 = call "Start_Initial.vi"("error in (no error)"=w526, "Reference"=w527) -> ("error out"=w522:errorcluster, "dup Reference"=w525:T7)  [unwired: 8 in]
            n524 = call "RunMacro.vi"("submacro"=TRUE, "error in (no error)"=w522, "Message_command"=w523, "queue"=w524) -> ("error out"=w519:errorcluster)  [unwired: 5 in, 2 out]
          }
        }
        "Current Line" <- w68
        n525 = local read "Cursor Position"() -> (w69:i32)
        n526 = Not Equal?(x=w69, y=w68) -> (x != y?=w67:bool)
        n527 = Unbundle By Name(w76) -> ("code"=w83:i32)
        n528 = And(x=w67, y="track \nseq.") -> (x .and. y?=w65:bool)
        n529 = case shown="True" w65 {
          tunnel: w62 -> [_ w106]
          frame False {
          }
          frame True {
            n530 = Generate User Event(user event=w106, event data cluster=TRUE ("event data")) -> ()  [unwired: 2 in, 2 out]
          }
        }
        n531 = Concatenate Strings(w72, w91) -> (→"Sequence Status":string)
        n532 = Not Equal To 0?(x=w83) -> (x != 0?=w75:bool)
        n533 = call <vilib>:"Clear Errors.vi"("error in (no error)"=w94) -> ("error out"=w78:errorcluster)  [unwired: 5 in, 1 out]
        n534 = property on="Error/\nwarning?" class="Bool (strict)"() -> ("Value"=w79:bool)  [unwired: 2 in, 2 out]
        n535 = property on="error \nindicator" class="Bool"("Visible"=w79) -> ()  [unwired: 2 in, 2 out]
        n536 = Or(x=w79, y=w75) -> (x .or. y?=w81:bool)
        n537 = Not(x="error \nindicator") -> (.not. x?=w80:bool)
        n538 = And(x=w81, y=w80) -> (x .and. y?=→"Error/\nwarning?":bool)
        n539 = case shown="True" w75 {
          tunnel: w76 -> [_ w107]
          frame False {
          }
          frame True {
            "most recent error" <- w107
          }
        }
        n540 = Wait Until Next ms Multiple(millisecond multiple="wait after each line executed (ms)") -> ()  [unwired: 1 out]
        "execution count" <- w85
      }
      n541 = Merge Errors(w51, w49) -> (w58:errorcluster)
    }
    frame Error {
    }
  }
  n542 = local write "sequence utility"(w1) -> ()
  n543 = local write "exec window"(w1) -> ()
  n544 = Unregister For Events(event registration refnum=w22, error in=w21) -> (error out=w20:errorcluster)
  n545 = Release Queue(queue=w23, error in (no error)=w20) -> (error out=w8:errorcluster)  [unwired: 1 in, 2 out]
  n546 = Destroy User Event(user event=w6, error in=w8) -> (error out=w7:errorcluster)
  n547 = Destroy User Event(user event=w5, error in=w7) -> ()  [unwired: 1 out]
  "Buffer History" <- w13
  "Buffer Edit" <- w13
